vi "app - monitor RUS scan -- works.vi"(10 "normalize phase":bool) -> ()   [LabVIEW 2015]
uses:
  complex region.ctl
  lorentzian.ctl
  circle corners.ctl
  cursor winow.ctl
  scale - offset gauge.ctl
  <vilib>/event_ctls.llb/eventvkey.ctl
  peak -- parameters -- complex fit.ctl
  wavepacket.ctl
  filter method control.ctl
  parameters -- scan monitor control.ctl
  monitor state.ctl
  peak monitor ctl - V2.ctl
  interpolation state - real.ctl
  countdown control.ctl
  cursor window action.ctl
  plot refs -- filter related.ctl
  monitor action.ctl
  read scan file control.ctl
  ctl -- name dispatcher -- action.ctl
  Q -- check range -- i -- real - window.vi
  array -- find interval - real.vi
  next chunk - read-write freq PID file - atomic actions .vi
  Q -- check range -- i -- integer.vi
  aggregator - vi - real - atomic.vi
  switch - C.vi
  acquire cursor window data.vi
  filter - complex - four.vi
  peak -- PM find lorenzian - V2.vi
  linear interp iiii- complex - z-omega.vi
  line -- complex.vi
  Q - not nan -- real.vi
  array -- find index - real.vi
  array -- interpolate -- i.vi
  Q - not nan -- integer.vi
  linear interpolation - real.vi
  tale of three indices.vi
  filter -- window span logic.vi
  linear interp iiii- complex - z-omega - divide.vi
  linear interpolation iiii- complex.vi
  containing bix.vi
  peak -- guess at omega -- dzdomega.vi
  <vilib>/Analysis/baseanly.llb/A x B.vi
  <vilib>/Analysis/baseanly.llb/Complex A x B.vi
  command stack.vi
  tale of three indices -- check state.vi
  peak -- z center from mult phase points.vi
  peak -- estimate for lorentzian.vi
  peak -- fake phase around center.vi
  peak -- get weights.vi
  peak -- four corner circle transformation logic.vi
  peak - fit phase around center - V1.vi
  circle center from three points.vi
  <vilib>/Utility/error.llb/Clear Errors.vi
  <vilib>/Utility/libraryn.llb/Check if File or Folder Exists.vi
  file -- read list of lines.vi
  parse -- find first line.vi
  parse -- get list of matches -- numbers.vi
  <vilib>/Utility/file.llb/Write To Spreadsheet File (string).vi
  <vilib>/gmath/function.llb/Binomial Coefficient.vi
  monitor -- write section files.vi
  <vilib>/Analysis/Matrix/Numeric/Conversions/Array To Matrix.vi
  <vilib>/Analysis/Matrix/Numeric/Conversions/Array To Matrix - RA2.vi
  <vilib>/Analysis/baseanly.llb/Inverse Matrix.vi
  <vilib>/Analysis/baseanly.llb/Real Inverse Matrix.vi
  array - generate range.vi
  peak -- fit function -- arctan.vi
  <vilib>/gmath/NumericalOptimization/Nonlinear Curve Fit.vi
  <vilib>/gmath/NumericalOptimization/Nonlinear Curve Fit LM.vi
  filter pipe - plot staff - more - V2.vi
panel:
  out "current resonance #":i32
  in  "overwriting !!":bool
  in  "current resonance #":i32
  in  "overwrite (d)":enum16{"DUMP", "WORK", ""}(ring)
  in  "Tab : monitor":enum32{"main", "EDIT"}(tab)
  in  "scan monitor control":T1={"gamma acc. frac. - min "=0.3, "gamma acc frac.. - max"=3.0, "peak acc. fraction (af)"=5.0, "min peak acc. window (kHz)"=0.5, "use"=enum."fraction", "abs gamma min(kHz)"=0.005, "abs gamma max(kHz)"=5.0, "# points"=5, "gamma-factor (fa)"=5.0, "interpolate"=enum."line", "init"=TRUE, "Unique strike parameters"=TRUE, "max peak acc. window (kHz)"=10.0, "spacing factor"=1.5, "iterate #"=1, "overwrite ctl?"=FALSE, "write _m files?"=FALSE, "max slope (kHz/sweep)"=0.5, "funnel state"=enum."funnel open"}
  in  "monitor state":T2={"header - gamma"=[], "header - frequency"=[], "# of peaks"=32, "peaks OK"=FALSE}
  in  "autopilot":enum32{"on", "off"}(tab)=enum."off"
  in  "timer \"v\"":dbl(slide)=3.8370000000122673 min=-14768275.999999998 max=2129711151.0 step=0.01 scale=0.0..5.0 scale format="%#3_3f"
  in  "timer  \"update\"":dbl(slide)=3.8469999999961146 min=-14763200.0 max=2129711151.0 step=0.010000000000000002 scale=0.0..10.0 scale format="%#3_3f"
  in  "Temperature (K)":dbl=300.461
  in  "Magn Field (T)":dbl
  in  "Array of states":T3[](array[typedef])=[{"delta"=-0.0016575432837271364, "gamma"=0.76553, "exp"=652.9113, "found?"=TRUE, "found"=652.9096424567163, "gamma found"=0.7013829844109373, "init linear"=FALSE, "interpolate"=enum."line", "gamma-factor"=5.0, "slope"=-0.0044851701449078974, "update freq?"=TRUE, "update gamma?"=TRUE, "acc factor"=5.0, "linear interpolation state"={"requested size"=5, "Array"=[652.9241022479541, 652.9241022479541, 652.9081701289798, 652.9081701289798, 652.9096424567163], "actual number of elements"=5}, "ind"=0.0, "gamma ratio"=0.9162057455761854, "gamma off limit?"=FALSE, "freq off limit?"=FALSE}, {"delta"=0.003759118773814407, "gamma"=0.17466, "exp"=1036.47326, "found?"=TRUE, "found"=1036.4770191187738, "gamma found"=0.18203135700796666, "init linear"=FALSE, "interpolate"=enum."line", "gamma-factor"=5.0, "slope"=-0.0007907161774346605, "update freq?"=TRUE, "update gamma?"=TRUE, "acc factor"=5.0, "linear interpolation state"={"requested size"=5, "Array"=[1036.4789192628243, 1036.4789192628243, 1036.4748123891509, 1036.4748123891509, 1036.4770191187738], "actual number of elements"=5}, "ind"=1.0, "gamma ratio"=1.042204036459216, "gamma off limit?"=FALSE, "freq off limit?"=FALSE}, {"delta"=0.0049091040252733364, "gamma"=0.2876, "exp"=1456.4571, "found?"=TRUE, "found"=1456.4620091040254, "gamma found"=0.29018960202050387, "init linear"=FALSE, "interpolate"=enum."line", "gamma-factor"=5.0, "slope"=0.0005201884449343197, "update freq?"=TRUE, "update gamma?"=TRUE, "acc factor"=5.0, "linear interpolation state"={"requested size"=5, "Array"=[1456.4592147196108, 1456.4592147196108, 1456.4588278352328, 1456.4588278352328, 1456.4620091040254], "actual number of elements"=5}, "ind"=2.0, "gamma ratio"=1.0090041794871483, "gamma off limit?"=FALSE, "freq off limit?"=FALSE}, {"delta"=0.0007394967815343989, "gamma"=0.09637, "exp"=1508.93353, "found?"=TRUE, "found"=1508.9342694967816, "gamma found"=0.09651911838128847, "init linear"=FALSE, "interpolate"=enum."line", "gamma-factor"=5.0, "slope"=-0.00010129910398973152, "update freq?"=TRUE, "update gamma?"=TRUE, "acc factor"=5.0, "linear interpolation state"={"requested size"=5, "Array"=[1508.934330293854, 1508.934330293854, 1508.9334388969608, 1508.9334388969608, 1508.9342694967816], "actual number of elements"=5}, "ind"=3.0, "gamma ratio"=1.0015473527164935, "gamma off limit?"=FALSE, "freq off limit?"=FALSE}, {"delta"=-0.029278381005497067, "gamma"=0.50061, "exp"=1568.62295, "found?"=TRUE, "found"=1568.5936716189944, "gamma found"=0.29241762919205017, "init linear"=FALSE, "interpolate"=enum."line", "gamma-factor"=5.0, "slope"=0.002435031997738406, "update freq?"=TRUE, "update gamma?"=TRUE, "acc factor"=5.0, "linear interpolation state"={"requested size"=5, "Array"=[1568.5938152073131, 1568.5938152073131, 1568.618452703927, 1568.618452703927, 1568.5936716189944], "actual number of elements"=5}, "ind"=4.0, "gamma ratio"=0.5841226287769924, "gamma off limit?"=FALSE, "freq off limit?"=FALSE}, {"delta"=0.0026202347487469524, "gamma"=0.0806, "exp"=1635.60553, "found?"=TRUE, "found"=1635.6081502347488, "gamma found"=0.08233227541925552, "init linear"=FALSE, "interpolate"=enum."line", "gamma-factor"=5.0, "slope"=-0.0002922362121171318, "update freq?"=TRUE, "update gamma?"=TRUE, "acc factor"=5.0, "linear interpolation state"={"requested size"=5, "Array"=[1635.6087113801916, 1635.6087113801916, 1635.6069113089588, 1635.6069113089588, 1635.6081502347488], "actual number of elements"=5}, "ind"=5.0, "gamma ratio"=1.0214922508592494, "gamma off limit?"=FALSE, "freq off limit?"=FALSE}, {"delta"=-0.002563017279953783, "gamma"=0.23948, "exp"=1764.33943, "found?"=TRUE, "found"=1764.33686698272, "gamma found"=0.24236340731954384, "init linear"=FALSE, "interpolate"=enum."line", "gamma-factor"=5.0, "slope"=-0.0006999494679621421, "update freq?"=TRUE, "update gamma?"=TRUE, "acc factor"=5.0, "linear interpolation state"={"requested size"=5, "Array"=[1764.3399842040806, 1764.3399842040806, 1764.339219152121, 1764.339219152121, 1764.33686698272], "actual number of elements"=5}, "ind"=6.0, "gamma ratio"=1.012040284447736, "gamma off limit?"=FALSE, "freq off limit?"=FALSE}, {"delta"=0.0013207520305513754, "gamma"=0.09629, "exp"=2205.10687, "found?"=TRUE, "found"=2205.1081907520306, "gamma found"=0.0924387831546914, "init linear"=FALSE, "interpolate"=enum."line", "gamma-factor"=5.0, "slope"=-7.088923128321767e-05, "update freq?"=TRUE, "update gamma?"=TRUE, "acc factor"=5.0, "linear interpolation state"={"requested size"=5, "Array"=[2205.108115975172, 2205.108115975172, 2205.1072575291464, 2205.1072575291464, 2205.1081907520306], "actual number of elements"=5}, "ind"=7.0, "gamma ratio"=0.9600039791742797, "gamma off limit?"=FALSE, "freq off limit?"=FALSE}, {"delta"=0.003409232488138514, "gamma"=0.15471, "exp"=2247.57115, "found?"=TRUE, "found"=2247.5745592324884, "gamma found"=0.1527741784741036, "init linear"=FALSE, "interpolate"=enum."line", "gamma-factor"=5.0, "slope"=-0.0009672962635522708, "update freq?"=TRUE, "update gamma?"=TRUE, "acc factor"=5.0, "linear interpolation state"={"requested size"=5, "Array"=[2247.5776758034717, 2247.5776758034717, 2247.574235982803, 2247.574235982803, 2247.5745592324884], "actual number of elements"=5}, "ind"=8.0, "gamma ratio"=0.9874874182283214, "gamma off limit?"=FALSE, "freq off limit?"=FALSE}, {"delta"=-0.008548894449631916, "gamma"=0.16479, "exp"=2285.77663, "found?"=TRUE, "found"=2285.76808110555, "gamma found"=0.1267187147828005, "init linear"=FALSE, "interpolate"=enum."line", "gamma-factor"=5.0, "slope"=-0.0016395337344147264, "update freq?"=TRUE, "update gamma?"=TRUE, "acc factor"=5.0, "linear interpolation state"={"requested size"=5, "Array"=[2285.7766292086317, 2285.7766292086317, 2285.77733007745, 2285.77733007745, 2285.76808110555], "actual number of elements"=5}, "ind"=9.0, "gamma ratio"=0.7689709010425421, "gamma off limit?"=FALSE, "freq off limit?"=FALSE}, {"delta"=0.0004447395758688799, "gamma"=0.21964, "exp"=2405.10472, "found?"=TRUE, "found"=2405.1051647395757, "gamma found"=0.22044726667002684, "init linear"=FALSE, "interpolate"=enum."line", "gamma-factor"=5.0, "slope"=-0.0008384914183989168, "update freq?"=TRUE, "update gamma?"=TRUE, "acc factor"=5.0, "linear interpolation state"={"requested size"=5, "Array"=[2405.1081612139637, 2405.1081612139637, 2405.10576924856, 2405.10576924856, 2405.1051647395757], "actual number of elements"=5}, "ind"=10.0, "gamma ratio"=1.0036754082590915, "gamma off limit?"=FALSE, "freq off limit?"=FALSE}, {"delta"=0.0003001280488206248, "gamma"=0.22537, "exp"=2483.53635, "found?"=TRUE, "found"=2483.5366501280487, "gamma found"=0.2213622002178064, "init linear"=FALSE, "interpolate"=enum."line", "gamma-factor"=5.0, "slope"=-5.884840269573033e-05, "update freq?"=TRUE, "update gamma?"=TRUE, "acc factor"=5.0, "linear interpolation state"={"requested size"=5, "Array"=[2483.536882570466, 2483.536882570466, 2483.5367589712696, 2483.5367589712696, 2483.5366501280487], "actual number of elements"=5}, "ind"=11.0, "gamma ratio"=0.9822168000080153, "gamma off limit?"=FALSE, "freq off limit?"=FALSE}, {"delta"=-0.00047377254441016703, "gamma"=0.1374, "exp"=2613.48596, "found?"=TRUE, "found"=2613.4854862274556, "gamma found"=0.13919976502630776, "init linear"=FALSE, "interpolate"=enum."line", "gamma-factor"=5.0, "slope"=-0.0004374731567804702, "update freq?"=TRUE, "update gamma?"=TRUE, "acc factor"=5.0, "linear interpolation state"={"requested size"=5, "Array"=[2613.4871697330486, 2613.4871697330486, 2613.4861620126653, 2613.4861620126653, 2613.4854862274556], "actual number of elements"=5}, "ind"=12.0, "gamma ratio"=1.0130987265379023, "gamma off limit?"=FALSE, "freq off limit?"=FALSE}, {"delta"=-0.0014333203166643216, "gamma"=0.23275, "exp"=2775.83282, "found?"=TRUE, "found"=2775.8313866796834, "gamma found"=0.2800873248387451, "init linear"=FALSE, "interpolate"=enum."line", "gamma-factor"=5.0, "slope"=9.053546469658613e-05, "update freq?"=TRUE, "update gamma?"=TRUE, "acc factor"=5.0, "linear interpolation state"={"requested size"=5, "Array"=[2775.8316113301, 2775.8316113301, 2775.8329659855785, 2775.8329659855785, 2775.8313866796834], "actual number of elements"=5}, "ind"=13.0, "gamma ratio"=1.2033827060740927, "gamma off limit?"=FALSE, "freq off limit?"=FALSE}, {"delta"=0.001513914386578108, "gamma"=0.0716, "exp"=2886.62499, "found?"=TRUE, "found"=2886.6265039143864, "gamma found"=0.07112662438840253, "init linear"=FALSE, "interpolate"=enum."line", "gamma-factor"=5.0, "slope"=-0.0006266225839499384, "update freq?"=TRUE, "update gamma?"=TRUE, "acc factor"=5.0, "linear interpolation state"={"requested size"=5, "Array"=[2886.628416499212, 2886.628416499212, 2886.6259754430316, 2886.6259754430316, 2886.6265039143864], "actual number of elements"=5}, "ind"=14.0, "gamma ratio"=0.9933886087765718, "gamma off limit?"=FALSE, "freq off limit?"=FALSE}, {"delta"=0.006262894615701953, "gamma"=0.14682, "exp"=2925.52376, "found?"=TRUE, "found"=2925.5300228946157, "gamma found"=0.14212049264176846, "init linear"=FALSE, "interpolate"=enum."line", "gamma-factor"=5.0, "slope"=-0.0013607249583583326, "update freq?"=TRUE, "update gamma?"=TRUE, "acc factor"=5.0, "linear interpolation state"={"requested size"=5, "Array"=[2925.5337999193525, 2925.5337999193525, 2925.5277467192377, 2925.5277467192377, 2925.5300228946157], "actual number of elements"=5}, "ind"=15.0, "gamma ratio"=0.9679913679455691, "gamma off limit?"=FALSE, "freq off limit?"=FALSE}, {"delta"=0.0008407358172917156, "gamma"=0.05724, "exp"=2968.74884, "found?"=TRUE, "found"=2968.7496807358175, "gamma found"=0.056604877858379594, "init linear"=FALSE, "interpolate"=enum."line", "gamma-factor"=5.0, "slope"=6.453693960793316e-05, "update freq?"=TRUE, "update gamma?"=TRUE, "acc factor"=5.0, "linear interpolation state"={"requested size"=5, "Array"=[2968.7492258726284, 2968.7492258726284, 2968.7489615156423, 2968.7489615156423, 2968.7496807358175], "actual number of elements"=5}, "ind"=16.0, "gamma ratio"=0.9889042253385674, "gamma off limit?"=FALSE, "freq off limit?"=FALSE}, {"delta"=0.0004893467435067578, "gamma"=0.18507, "exp"=3117.27562, "found?"=TRUE, "found"=3117.2761093467434, "gamma found"=0.18508310581473786, "init linear"=FALSE, "interpolate"=enum."line", "gamma-factor"=5.0, "slope"=-0.000674382079159841, "update freq?"=TRUE, "update gamma?"=TRUE, "acc factor"=5.0, "linear interpolation state"={"requested size"=5, "Array"=[3117.278479994366, 3117.278479994366, 3117.27647746882, 3117.27647746882, 3117.2761093467434], "actual number of elements"=5}, "ind"=17.0, "gamma ratio"=1.0000708154467923, "gamma off limit?"=FALSE, "freq off limit?"=FALSE}, {"delta"=0.0009432243264200224, "gamma"=0.11467, "exp"=3141.4319, "found?"=TRUE, "found"=3141.4328432243265, "gamma found"=0.11506466086057514, "init linear"=FALSE, "interpolate"=enum."line", "gamma-factor"=5.0, "slope"=-0.0002722086093854159, "update freq?"=TRUE, "update gamma?"=TRUE, "acc factor"=5.0, "linear interpolation state"={"requested size"=5, "Array"=[3141.4337316093643, 3141.4337316093643, 3141.432786293347, 3141.432786293347, 3141.4328432243265], "actual number of elements"=5}, "ind"=18.0, "gamma ratio"=1.0034417097808943, "gamma off limit?"=FALSE, "freq off limit?"=FALSE}, {"delta"=0.006890674223541282, "gamma"=0.19401, "exp"=3268.65403, "found?"=TRUE, "found"=3268.6609206742237, "gamma found"=0.1947000973954296, "init linear"=FALSE, "interpolate"=enum."line", "gamma-factor"=5.0, "slope"=0.001370561413350515, "update freq?"=TRUE, "update gamma?"=TRUE, "acc factor"=5.0, "linear interpolation state"={"requested size"=5, "Array"=[3268.654487682439, 3268.654487682439, 3268.6553273130035, 3268.6553273130035, 3268.6609206742237], "actual number of elements"=5}, "ind"=19.0, "gamma ratio"=1.0035570197176928, "gamma off limit?"=FALSE, "freq off limit?"=FALSE}, {"delta"=-0.00036122355459156097, "gamma"=0.09375, "exp"=3447.74234, "found?"=TRUE, "found"=3447.741978776445, "gamma found"=0.09343849466512388, "init linear"=FALSE, "interpolate"=enum."line", "gamma-factor"=5.0, "slope"=-0.0002539216459263116, "update freq?"=TRUE, "update gamma?"=TRUE, "acc factor"=5.0, "linear interpolation state"={"requested size"=5, "Array"=[3447.7428802682552, 3447.7428802682552, 3447.742144035429, 3447.742144035429, 3447.741978776445], "actual number of elements"=5}, "ind"=20.0, "gamma ratio"=0.9966772764279881, "gamma off limit?"=FALSE, "freq off limit?"=FALSE}, {"delta"=-3486.5123, "gamma"=0.01485, "exp"=3486.5123, "found?"=FALSE, "found"=0.0, "gamma found"=0.0, "init linear"=TRUE, "interpolate"=enum."line", "gamma-factor"=5.0, "slope"=0.0, "update freq?"=FALSE, "update gamma?"=FALSE, "acc factor"=5.0, "linear interpolation state"={"requested size"=5, "Array"=[0.0, 0.0, 0.0, 0.0, 3486.5122984940626], "actual number of elements"=1}, "ind"=21.0, "gamma ratio"=0.0, "gamma off limit?"=TRUE, "freq off limit?"=TRUE}, {"delta"=0.005188108485072007, "gamma"=0.2862, "exp"=3737.75053, "found?"=TRUE, "found"=3737.755718108485, "gamma found"=0.25947921890028686, "init linear"=FALSE, "interpolate"=enum."line", "gamma-factor"=5.0, "slope"=-0.0006564744841307402, "update freq?"=TRUE, "update gamma?"=TRUE, "acc factor"=5.0, "linear interpolation state"={"requested size"=5, "Array"=[3737.7568178710067, 3737.7568178710067, 3737.752452651206, 3737.752452651206, 3737.755718108485], "actual number of elements"=5}, "ind"=22.0, "gamma ratio"=0.9066359849765439, "gamma off limit?"=FALSE, "freq off limit?"=FALSE}, {"delta"=0.05791749378431632, "gamma"=0.1209, "exp"=3773.78708, "found?"=FALSE, "found"=3773.8449974937844, "gamma found"=0.0018969298658040622, "init linear"=FALSE, "interpolate"=enum."line", "gamma-factor"=7.0, "slope"=-0.027493364620750072, "update freq?"=TRUE, "update gamma?"=TRUE, "acc factor"=7.0, "linear interpolation state"={"requested size"=5, "Array"=[0.0, 3773.880271706499, 3773.8206547185614, 3773.825284977259, 3773.7870837381997], "actual number of elements"=4}, "ind"=23.0, "gamma ratio"=0.015690073331712674, "gamma off limit?"=TRUE, "freq off limit?"=FALSE}, {"delta"=0.0016448427732029813, "gamma"=0.14541, "exp"=4176.53307, "found?"=TRUE, "found"=4176.534714842774, "gamma found"=0.14055145401454877, "init linear"=FALSE, "interpolate"=enum."line", "gamma-factor"=5.0, "slope"=0.001082140458165668, "update freq?"=TRUE, "update gamma?"=TRUE, "acc factor"=5.0, "linear interpolation state"={"requested size"=5, "Array"=[4176.530918624351, 4176.530918624351, 4176.534147592093, 4176.534147592093, 4176.534714842774], "actual number of elements"=5}, "ind"=24.0, "gamma ratio"=0.9665872636995307, "gamma off limit?"=FALSE, "freq off limit?"=FALSE}, {"delta"=0.006093070963288483, "gamma"=0.07631, "exp"=4238.40966, "found?"=TRUE, "found"=4238.415753070964, "gamma found"=0.07370934433890397, "init linear"=FALSE, "interpolate"=enum."line", "gamma-factor"=5.0, "slope"=-0.0001927513594273478, "update freq?"=TRUE, "update gamma?"=TRUE, "acc factor"=5.0, "linear interpolation state"={"requested size"=5, "Array"=[4238.415194475135, 4238.415194475135, 4238.412149769886, 4238.412149769886, 4238.415753070964], "actual number of elements"=5}, "ind"=25.0, "gamma ratio"=0.9659198576713925, "gamma off limit?"=FALSE, "freq off limit?"=FALSE}, {"delta"=0.0014712240090375417, "gamma"=0.10797, "exp"=4931.57573, "found?"=TRUE, "found"=4931.577201224009, "gamma found"=0.1106825599113035, "init linear"=FALSE, "interpolate"=enum."line", "gamma-factor"=5.0, "slope"=0.0010064907773630694, "update freq?"=TRUE, "update gamma?"=TRUE, "acc factor"=5.0, "linear interpolation state"={"requested size"=5, "Array"=[4931.573629158262, 4931.573629158262, 4931.5765499345425, 4931.5765499345425, 4931.577201224009], "actual number of elements"=5}, "ind"=26.0, "gamma ratio"=1.0251232741622998, "gamma off limit?"=FALSE, "freq off limit?"=FALSE}, {"delta"=0.01094153662052122, "gamma"=0.05188, "exp"=5475.82656, "found?"=TRUE, "found"=5475.837501536621, "gamma found"=0.11863591544266465, "init linear"=FALSE, "interpolate"=enum."line", "gamma-factor"=8.0, "slope"=0.0012847163761034609, "update freq?"=TRUE, "update gamma?"=TRUE, "acc factor"=8.0, "linear interpolation state"={"requested size"=5, "Array"=[5475.831455900791, 5475.831455900791, 5475.832211792886, 5475.832211792886, 5475.837501536621], "actual number of elements"=5}, "ind"=27.0, "gamma ratio"=2.2867369977383314, "gamma off limit?"=FALSE, "freq off limit?"=FALSE}, {"delta"=-5768.35916, "gamma"=0.005, "exp"=5768.35916, "found?"=FALSE, "found"=0.0, "gamma found"=0.0, "init linear"=TRUE, "interpolate"=enum."line", "gamma-factor"=5.0, "slope"=0.0, "update freq?"=FALSE, "update gamma?"=FALSE, "acc factor"=5.0, "linear interpolation state"={"requested size"=5, "Array"=[0.0, 0.0, 0.0, 0.0, 5768.359158074293], "actual number of elements"=1}, "ind"=28.0, "gamma ratio"=0.0, "gamma off limit?"=TRUE, "freq off limit?"=TRUE}, {"delta"=18.256138418231785, "gamma"=0.02905, "exp"=6148.70194, "found?"=FALSE, "found"=6166.958078418232, "gamma found"=4.5314912463139816e-05, "init linear"=TRUE, "interpolate"=enum."line", "gamma-factor"=5.0, "slope"=0.0, "update freq?"=FALSE, "update gamma?"=FALSE, "acc factor"=5.0, "linear interpolation state"={"requested size"=5, "Array"=[0.0, 0.0, 0.0, 0.0, 6148.701943422434], "actual number of elements"=1}, "ind"=29.0, "gamma ratio"=0.001559893716459202, "gamma off limit?"=TRUE, "freq off limit?"=TRUE}, {"delta"=0.004358224254247034, "gamma"=0.0424, "exp"=5751.24344, "found?"=TRUE, "found"=5751.247798224254, "gamma found"=0.0686871247901866, "init linear"=TRUE, "interpolate"=enum."line", "gamma-factor"=7.0, "slope"=0.0, "update freq?"=FALSE, "update gamma?"=FALSE, "acc factor"=7.0, "linear interpolation state"={"requested size"=5, "Array"=[0.0, 0.0, 0.0, 0.0, 5751.24344], "actual number of elements"=1}, "ind"=30.0, "gamma ratio"=1.619979358259118, "gamma off limit?"=FALSE, "freq off limit?"=FALSE}, {"delta"=0.02459476473813993, "gamma"=0.14229, "exp"=6300.95565, "found?"=TRUE, "found"=6300.980244764738, "gamma found"=0.1593322314931949, "init linear"=FALSE, "interpolate"=enum."line", "gamma-factor"=7.0, "slope"=0.001076212803600356, "update freq?"=TRUE, "update gamma?"=TRUE, "acc factor"=7.0, "linear interpolation state"={"requested size"=5, "Array"=[6300.9711810739645, 6300.9711810739645, 6300.963815820454, 6300.963815820454, 6300.980244764738], "actual number of elements"=5}, "ind"=31.0, "gamma ratio"=1.1197711117660756, "gamma off limit?"=FALSE, "freq off limit?"=FALSE}]
  in  "dump/work NEW (\"n\")":enum16{"DUMP", "WORK", ""}(ring)
  in  "NEW freq":dbl[](array[numeric])=[652.901381931682, 1036.4745243360126, 1456.4611794080774, 1508.93365767837, 1568.6109465842878, 1635.607002413974, 1764.33695489062, 2205.1075748844396, 2247.5727746722177, 2285.770281334339, 2405.104089658669, 2483.536610097096, 2613.485117524306, 2775.8323798686024, 2886.625177692022, 2925.5265410594843, 2968.74940471329, 3117.275181708386, 3141.432359180121, 3268.6602218172616, 3447.7416437118245, 3486.5122984940626, 3737.7528824071287, 3773.7595903735782, 4176.536215876507, 4238.4135100581225, 4931.5785313542565, 5475.8368215339215, 5768.359158074293, 6148.701943422434, 5751.24344, 6300.973276349126]
  in  "NEW gamma":dbl[](array[numeric])=[0.7013829844109373, 0.18203135700796666, 0.29018960202050387, 0.09651911838128847, 0.29241762919205017, 0.08233227541925552, 0.24236340731954384, 0.0924387831546914, 0.1527741784741036, 0.1267187147828005, 0.22044726667002684, 0.2213622002178064, 0.13919976502630776, 0.2800873248387451, 0.07112662438840253, 0.14212049264176846, 0.056604877858379594, 0.18508310581473786, 0.11506466086057514, 0.1947000973954296, 0.09343849466512388, 0.01485, 0.25947921890028686, 0.1209, 0.14055145401454877, 0.07370934433890397, 0.1106825599113035, 0.11863591544266465, 0.005, 0.02905, 0.0424, 0.1593322314931949]
  in  "OLD gamma":dbl[](array[numeric])
  in  "OLD freq":dbl[](array[numeric])
  out "cp lorentzian":T5={"Amplitude"=0.000340055891053764, "omega(0)"=3392.560000065714, "Gamma"=11.91999763250351, "phase"=1.0574274315248449, "Q"=284.61079478865537, "Norm  Ampl"=nan, "z (inf)"=-2.2995916620324662e-05-1.1031702558117846e-05i, "4corners"={"z (-pi/2)"=1.5865449989673634e-05-1.9155492294065609e-07i, "z(inf)"=-2.2995916620324662e-05-1.1031702558117846e-05i, "z (pi/2)"=-1.2155768985147472e-05-4.9893069168116145e-05i, "z center"=1.8548405022630806e-06-2.50423120455284e-05i, "z(0)"=2.6705597624850824e-05-3.905292153293895e-05i, "radius"=2.8528184445817156e-05}} {"z (inf)" format="%#9_9f"; "Q" format="%#9_9f"; "phase" format="%#9_9f"; "Gamma" format="%#9_9f"; "omega(0)" format="%#9_9f"}
  out "index":i32[](array[numeric])=[0, 1, 2, 3, 4, 5, 6, 7, 8, 9, 10, 11, 12, 13, 14, 15, 16, 17, 18, 19, 20, 21, 22, 23, 24, 25, 26, 27, 28, 29, 30, 31, 32, 33, 34, 35, 36, 37, 38, 39, 40, 41, 42, 43, 44, 45, 46, 47, 48, 49, 50, 51, 52, 53, 54, 55, 56, 57, 58, 59, 60, 61, 62, 63, 64, 65, 66, 67, 68, 69, 70, 71, 72, 73, 74, 75, 76, 77, 78, 79, 80, 81, 82, 83, 84, 85, 86, 87, 88, 89, 90, 91, 92, 93, 94, 95, 96, 97, 98, 99]
  in  "Tab : everything":T7(tab)
  in  "Tab :  Fit controls":enum32{"complex plane", "complex plane 2"}(tab)
  in  "Plot: fragment - filter":cluster{dbl[], dbl[]}[](graph)=[{array[953 elements], array[953 elements]}, {array[953 elements], array[953 elements]}, {array[953 elements], array[953 elements]}, {array[953 elements], array[953 elements]}]
  in  "scale gauge: Plot: complex plane - filter":dbl(slide)=0.00199 min=0.0 max=0.3 step=1e-05 scale=0.0001..0.3 scale format="%#_5g"
  in  "Plot: complex plane - filter":cluster{dbl[], dbl[]}[](graph)=[{array[953 elements], array[953 elements]}, {array[953 elements], array[953 elements]}, {[6.147901040838566e-05, 6.135373133876665e-05, 6.097838854916284e-05, 6.0354463346086974e-05, 5.948441807727129e-05, 5.837168641390595e-05, 5.702065979950748e-05, 5.54366701188976e-05, 5.362596865568959e-05, 5.1595701421327945e-05, 4.9353880953045816e-05, 4.690935469204115e-05, 4.427177006666834e-05, 4.145153641844591e-05, 3.8459783921141216e-05, 3.5308319655059415e-05, 3.200958100989166e-05, 2.8576586600020083e-05, 2.5022884885994518e-05, 2.1362500704948304e-05, 1.7609879920973602e-05, 1.3779832413895373e-05, 9.887473631441806e-06, 5.948164935477676e-06, 1.9774529777269755e-06, -2.0089916557587785e-06, -5.995436289244519e-06, -9.96614824699522e-06, -1.3905456942959363e-05, -1.779781572541292e-05, -2.1627863232491146e-05, -2.5380484016465848e-05, -2.904086819751206e-05, -3.259456991153764e-05, -3.6027564321409215e-05, -3.932630296657695e-05, -4.247776723265876e-05, -4.5469519729963454e-05, -4.8289753378185884e-05, -5.09273380035587e-05, -5.3371864264563346e-05, -5.561368473284548e-05, -5.764395196720713e-05, -5.945465343041514e-05, -6.103864311102503e-05, -6.238966972542349e-05, -6.350240138878883e-05, -6.437244665760451e-05, -6.499637186068038e-05, -6.537171465028419e-05, -6.54969937199032e-05, -6.537171465028419e-05, -6.499637186068038e-05, -6.437244665760451e-05, -6.350240138878883e-05, -6.238966972542349e-05, -6.103864311102501e-05, -5.945465343041513e-05, -5.764395196720712e-05, -5.5613684732845474e-05, -5.337186426456334e-05, -5.092733800355868e-05, -4.828975337818588e-05, -4.546951972996345e-05, -4.2477767232658746e-05, -3.9326302966576966e-05, -3.602756432140918e-05, -3.2594569911537626e-05, -2.904086819751202e-05, -2.5380484016465838e-05, -2.1627863232491146e-05, -1.7797815725412892e-05, -1.390545694295935e-05, -9.966148246995179e-06, -5.995436289244506e-06, -2.0089916557587802e-06, 1.9774529777270017e-06, 5.9481649354776745e-06, 9.887473631441845e-06, 1.3779832413895386e-05, 1.760987992097359e-05, 2.1362500704948328e-05, 2.5022884885994515e-05, 2.8576586600020124e-05, 3.200958100989167e-05, 3.5308319655059456e-05, 3.8459783921141236e-05, 4.145153641844591e-05, 4.427177006666836e-05, 4.690935469204116e-05, 4.9353880953045836e-05, 5.159570142132796e-05, 5.362596865568959e-05, 5.543667011889761e-05, 5.702065979950749e-05, 5.837168641390596e-05, 5.9484418077271304e-05, 6.0354463346086974e-05, 6.097838854916284e-05, 6.135373133876665e-05], [-1.1205323218261426e-05, -7.218878584775678e-06, -3.2481666270249814e-06, 6.911420689391552e-07, 4.583500851392718e-06, 8.413548358470941e-06, 1.2166169142445653e-05, 1.5826553323491864e-05, 1.938025503751744e-05, 2.2813249447389007e-05, 2.6111988092556765e-05, 2.9263452358638565e-05, 3.225520485594326e-05, 3.507543850416568e-05, 3.7713023129538496e-05, 4.015754939054316e-05, 4.239936985882529e-05, 4.442963709318694e-05, 4.6240338556394946e-05, 4.782432823700483e-05, 4.917535485140329e-05, 5.028808651476863e-05, 5.115813178358432e-05, 5.178205698666018e-05, 5.2157399776263995e-05, 5.2282678845883e-05, 5.2157399776263995e-05, 5.178205698666017e-05, 5.115813178358432e-05, 5.028808651476863e-05, 4.917535485140329e-05, 4.7824328237004825e-05, 4.624033855639494e-05, 4.4429637093186926e-05, 4.239936985882528e-05, 4.015754939054316e-05, 3.7713023129538496e-05, 3.5075438504165676e-05, 3.2255204855943246e-05, 2.926345235863855e-05, 2.611198809255677e-05, 2.2813249447389007e-05, 1.9380255037517432e-05, 1.5826553323491847e-05, 1.216616914244564e-05, 8.413548358470924e-06, 4.583500851392722e-06, 6.911420689391518e-07, -3.2481666270249915e-06, -7.218878584775692e-06, -1.1205323218261446e-05, -1.5191767851747172e-05, -1.9162479809497872e-05, -2.3101788505462016e-05, -2.6994147287915587e-05, -3.082419479499382e-05, -3.4576815578968526e-05, -3.8237199760014716e-05, -4.179090147404029e-05, -4.5223895883911866e-05, -4.852263452907963e-05, -5.167409879516143e-05, -5.466585129246611e-05, -5.7486084940688535e-05, -6.0123669566061355e-05, -6.2568195827066e-05, -6.481001629534815e-05, -6.684028352970978e-05, -6.865098499291781e-05, -7.023497467352768e-05, -7.158600128792615e-05, -7.26987329512915e-05, -7.356877822010717e-05, -7.419270342318303e-05, -7.456804621278685e-05, -7.469332528240585e-05, -7.456804621278685e-05, -7.419270342318303e-05, -7.356877822010717e-05, -7.269873295129148e-05, -7.158600128792615e-05, -7.023497467352767e-05, -6.86509849929178e-05, -6.684028352970978e-05, -6.481001629534813e-05, -6.256819582706598e-05, -6.0123669566061334e-05, -5.7486084940688535e-05, -5.4665851292466084e-05, -5.167409879516141e-05, -4.8522634529079576e-05, -4.522389588391184e-05, -4.179090147404029e-05, -3.823719976001468e-05, -3.45768155789685e-05, -3.0824194794993756e-05, -2.6994147287915553e-05, -2.310178850546201e-05, -1.9162479809497842e-05, -1.5191767851747167e-05]}, {[2.180843613001339e-05, -2.008991706602334e-06, -8.45318187396811e-06], [2.015688719802568e-05, -1.1205323149030123e-05, 1.4773194307782804e-05]}, {[3.113757403751932e-06, 2.0471841396985487e-06, 9.806108756451657e-07, -8.596238840821741e-08, -1.1525356524616005e-06, -2.2191089165149835e-06, -3.2856821805683666e-06, -4.35225544462175e-06, -5.418828708675133e-06, -6.485401972728517e-06, -7.551975236781899e-06, -8.618548500835281e-06, -9.685121764888665e-06, -1.0751695028942049e-05, -1.1818268292995431e-05, -1.2884841557048813e-05, -1.3951414821102197e-05, -1.5017988085155581e-05, -1.6084561349208965e-05, -1.7151134613262346e-05], [7.143908232533313e-06, 6.9167218796742506e-06, 6.689535526815188e-06, 6.462349173956126e-06, 6.235162821097064e-06, 6.0079764682380015e-06, 5.780790115378939e-06, 5.553603762519877e-06, 5.326417409660815e-06, 5.0992310568017525e-06, 4.87204470394269e-06, 4.644858351083628e-06, 4.417671998224566e-06, 4.1904856453655035e-06, 3.963299292506441e-06, 3.736112939647379e-06, 3.5089265867883167e-06, 3.2817402339292544e-06, 3.054553881070192e-06, 2.82736752821113e-06]}, {[-2.0089917066023344e-06, -9.360762157193256e-07, 1.3683927516368315e-07, 1.2097547660466921e-06, 2.2826702569297007e-06, 3.3555857478127092e-06, 4.428501238695719e-06, 5.501416729578727e-06, 6.574332220461736e-06, 7.647247711344744e-06, 8.720163202227753e-06, 9.793078693110761e-06, 1.0865994183993772e-05, 1.193890967487678e-05, 1.3011825165759789e-05, 1.4084740656642797e-05, 1.5157656147525806e-05, 1.6230571638408814e-05, 1.7303487129291823e-05, 1.837640262017483e-05], [-1.1205323149030123e-05, -1.1205323149030123e-05, -1.1205323149030123e-05, -1.1205323149030123e-05, -1.1205323149030123e-05, -1.1205323149030123e-05, -1.1205323149030123e-05, -1.1205323149030123e-05, -1.1205323149030123e-05, -1.1205323149030123e-05, -1.1205323149030123e-05, -1.1205323149030123e-05, -1.1205323149030123e-05, -1.1205323149030123e-05, -1.1205323149030123e-05, -1.1205323149030123e-05, -1.1205323149030123e-05, -1.1205323149030123e-05, -1.1205323149030123e-05, -1.1205323149030123e-05]}]
  out "Plot: dz/domega":cluster{"omega out":dbl[], dbl[]}(graph)
  out "Plot: win omega":T8(graph)
  out "Plot: phase":cluster{"omega out":dbl[], dbl[]}(graph)
  out "Plot: phase around center":cluster{dbl[], dbl[]}[](graph)
  out "Plot: fragment":cluster{dbl[], dbl[]}[](graph)
  out "Plot: complex plane":cluster{dbl[], dbl[]}[](graph)=[{array[953 elements], array[953 elements]}, {[3.0383024948080237e-05, 3.01580716927693e-05, 2.9486759574053305e-05, 2.8379675585066826e-05, 2.68542791016561e-05, 2.4934626537592202e-05, 2.2650991960555277e-05, 2.0039389652002364e-05, 1.714100614043495e-05, 1.4001550665240835e-05, 1.0670534314683625e-05, 7.200489206464318e-06, 3.646140024844015e-06, 6.354097968214359e-08, -3.4908082019381657e-06, -6.960853310157466e-06, -1.0291869660714675e-05, -1.3431325135908794e-05, -1.6329708647476206e-05, -1.8941310956029118e-05, -2.1224945533066037e-05, -2.314459809712994e-05, -2.4669994580540667e-05, -2.5777078569527143e-05, -2.6448390688243138e-05, -2.6673343943554075e-05, -2.6448390688243138e-05, -2.5777078569527143e-05, -2.466999458054066e-05, -2.3144598097129935e-05, -2.1224945533066034e-05, -1.8941310956029115e-05, -1.63297086474762e-05, -1.343132513590878e-05, -1.0291869660714658e-05, -6.960853310157466e-06, -3.49080820193816e-06, 6.354097968214909e-08, 3.646140024844027e-06, 7.200489206464335e-06, 1.0670534314683618e-05, 1.4001550665240833e-05, 1.7141006140434956e-05, 2.003938965200237e-05, 2.2650991960555284e-05, 2.4934626537592213e-05, 2.68542791016561e-05, 2.837967558506683e-05, 2.948675957405331e-05, 3.01580716927693e-05], [-2.50423120455284e-05, -2.1466782441215247e-05, -1.7947641074679964e-05, -1.454038690750597e-05, -1.1298754373304577e-05, -8.273865953597556e-06, -5.513425945744431e-06, -3.060968137675989e-06, -9.551692540527458e-07, 7.707609987872854e-07, 2.0896036697360487e-06, 2.9805598220342752e-06, 3.429578544928799e-06, 3.429578544928799e-06, 2.980559822034272e-06, 2.0896036697360487e-06, 7.70760998787282e-07, -9.551692540527492e-07, -3.060968137675989e-06, -5.513425945744438e-06, -8.273865953597552e-06, -1.129875437330458e-05, -1.4540386907505977e-05, -1.7947641074679964e-05, -2.146678244121525e-05, -2.504231204552841e-05, -2.8617841649841554e-05, -3.213698301637684e-05, -3.554423718355084e-05, -3.878586971775222e-05, -4.1810758137459246e-05, -4.4571198145312364e-05, -4.702365595338081e-05, -4.912945483700406e-05, -5.085538508984409e-05, -5.217422776079284e-05, -5.3065183913091077e-05, -5.35142026359856e-05, -5.35142026359856e-05, -5.306518391309107e-05, -5.217422776079285e-05, -5.085538508984409e-05, -4.912945483700405e-05, -4.7023655953380806e-05, -4.457119814531235e-05, -4.181075813745923e-05, -3.878586971775222e-05, -3.5544237183550826e-05, -3.213698301637683e-05, -2.8617841649841537e-05]}, {[-2.2995916620324662e-05, -2.051084090806589e-05, -1.8025765195807113e-05, -1.554068948354834e-05, -1.3055613771289565e-05, -1.057053805903079e-05, -8.085462346772018e-06, -5.600386634513241e-06, -3.1153109222544683e-06, -6.302352099956953e-07, 1.854840502263081e-06, 4.339916214521854e-06, 6.824991926780627e-06, 9.310067639039403e-06, 1.179514335129818e-05, 1.4280219063556949e-05, 1.6765294775815725e-05, 1.92503704880745e-05, 2.173544620033327e-05, 2.4220521912592048e-05], [-1.1031702558117846e-05, -1.2432763506858901e-05, -1.3833824455599956e-05, -1.5234885404341013e-05, -1.6635946353082066e-05, -1.8037007301823124e-05, -1.943806825056418e-05, -2.0839129199305234e-05, -2.224019014804629e-05, -2.3641251096787344e-05, -2.50423120455284e-05, -2.6443372994269454e-05, -2.7844433943010512e-05, -2.9245494891751567e-05, -3.064655584049262e-05, -3.2047616789233674e-05, -3.344867773797473e-05, -3.484973868671579e-05, -3.625079963545684e-05, -3.7651860584197894e-05]}, {[1.5865449989673634e-05, 1.4464389040932579e-05, 1.3063328092191524e-05, 1.1662267143450467e-05, 1.0261206194709412e-05, 8.860145245968358e-06, 7.459084297227301e-06, 6.058023348486246e-06, 4.656962399745191e-06, 3.255901451004136e-06, 1.854840502263081e-06, 4.5377955352202603e-07, -9.472813952190323e-07, -2.3483423439600873e-06, -3.7494032927011422e-06, -5.150464241442197e-06, -6.551525190183252e-06, -7.952586138924307e-06, -9.353647087665362e-06, -1.0754708036406417e-05], [-1.9155492294065947e-07, -2.6766306351994337e-06, -5.161706347458208e-06, -7.646782059716982e-06, -1.0131857771975756e-05, -1.2616933484234531e-05, -1.5102009196493304e-05, -1.758708490875208e-05, -2.0072160621010853e-05, -2.2557236333269626e-05, -2.5042312045528402e-05, -2.7527387757787175e-05, -3.0012463470045948e-05, -3.2497539182304725e-05, -3.49826148945635e-05, -3.746769060682227e-05, -3.995276631908105e-05, -4.243784203133982e-05, -4.492291774359859e-05, -4.740799345585737e-05]}, {[0.04673210164257447, 0.049919815487102684, 0.05307633107191166, 0.056199675677509844, 0.05928789731518806, 0.06233906594694866, 0.06535127469171664, 0.06832264101707818, 0.07125130791580202, 0.0741354450664087, 0.07697324997706184, 0.07976294911206679, 0.0825027990002728, 0.0851910873246857, 0.08782613399261033, 0.09040629218565366, 0.09292994938893286, 0.09539552839884442, 0.09780148830876523, 0.10014632547206899], [-0.12810601858774873, -0.1268978066952708, -0.12561028780431027, -0.1242442665722635, -0.12280059671793454, -0.12128018048798891, -0.11968396809307863, -0.11801295711399153, -0.11626819187819583, -0.11445076280716932, -0.11256180573492151, -0.11060250119813439, -0.10857407369836529, -0.10647779093677343, -0.10431496302184781, -0.10208694165063226, -0.09979511926395848, -0.09744092817621612, -0.09502583968020283, -0.09255136312761404]}, {[0.05358614321681127, 0.05724138842520362, 0.06086085962911791, 0.0644422947768705, 0.06798345558807486, 0.07148212895249367, 0.07493612831316095, 0.07834329503290884, 0.08170149974344551, 0.08500864367614118, 0.08826265997369011, 0.09146151498182913, 0.09460320952030535, 0.09768578013229881, 0.10070730031151905, 0.10366588170620873, 0.1065596752993022, 0.1093868725640008, 0.11214570659404333, 0.11483445320796498], [-0.1468949013139417, -0.145509485010567, -0.14403313001559898, -0.142466759002852, -0.14081135090322142, -0.13906794029288377, -0.13723761674671997, -0.13532152415736678, -0.13332086002032104, -0.13123687468554396, -0.12907087057603317, -0.1268242013738506, -0.12449827117411537, -0.12209453360749002, -0.11961449093170867, -0.11705969309271483, -0.11443173675599556, -0.11173226430871766, -0.10896296283328909, -0.10612556305298726]}, {array[953 elements], array[953 elements]}]
  in  "scale gauge: Plot: complex plane":dbl(slide)=0.08418000000000002 min=0.0 max=0.3 step=1e-05 scale=0.0001..1.0 scale format="%#_2g"
  in  "plot staff":enum16{"plot", "do not plot", "a"}(ring)=enum."do not plot"
  out "pm lorentzian":T5={"Amplitude"=0.000340055891053764, "omega(0)"=3392.560000065714, "Gamma"=11.91999763250351, "phase"=1.0574274315248449, "Q"=284.61079478865537, "Norm  Ampl"=nan, "z (inf)"=-2.2995916620324662e-05-1.1031702558117846e-05i, "4corners"={"z (-pi/2)"=1.5865449989673634e-05-1.9155492294065609e-07i, "z(inf)"=-2.2995916620324662e-05-1.1031702558117846e-05i, "z (pi/2)"=-1.2155768985147472e-05-4.9893069168116145e-05i, "z center"=1.8548405022630806e-06-2.50423120455284e-05i, "z(0)"=2.6705597624850824e-05-3.905292153293895e-05i, "radius"=2.8528184445817156e-05}} {"z (inf)" format="%#9_9f"; "Q" format="%#9_9f"; "phase" format="%#9_9f"; "Gamma" format="%#9_9f"; "omega(0)" format="%#9_9f"}
  in  "use fast fit?":bool=TRUE
  out "window width (kHz)":dbl=76.27809365793496
  out "window center (kHz)":dbl=3399.029286744401
  out "# of points in window":dbl=953.475933538175
  in  "Tab : all plot":enum32{"Page 1"}(tab)
  in  "scale gauge : All plot":T9={"scale offset"=0.5005000000000001, "scale range"=0.019950000000000002} {"scale range" min=0.0 max=1.0 step=1e-05 scale=0.001..1.0 scale format="%#_2g"; "scale offset" min=0.0 max=1.0 step=1e-05 scale=0.001..1.0 scale format="%#_2g"}
  out "Plot: All":cluster{"all rows":dbl[], "all rows":dbl[]}[](graph)
  in  "Sweep folder path":path=path "C:/data/Ultrasound/birdcage/Hg1201/Test"
  out "scan file found":bool=TRUE
  in  "source":enum16{"last scan file", "manual"}(ring)
  in  "subtract linear BG":bool
  out "complex region":T10={"max re"=1.5, "min re"=-1.5, "max im"=1.5, "min im"=-1.5, "delta re"=3.0, "delta im"=3.0, "center re"=0.0, "delta  z"=3.0+3.0i, "center im"=0.0, "center z"=0.0+0.0i, "d im"=0.0, "d re"=0.0, "d z"=0.0+0.0i}
  in  "cursor bracket: All, data window":T11={"left"=3360.8902399154335, "right "=3437.1683335733683, "center"=3399.029286744401, "window"=76.27809365793496, "cursors"=[0, 1, 2], "relative"=0, "absolute"=0, "fixed vertical offset"=0.0, "vertical offset"=0.0, "skew"=0.0, "default window frac"=0.1, "kind"=enum."symmetric", "skew.left"=0.5, "skew.right"=0.5, "Plot ref"=refnum, "wing order"=enum."forw"}
  out "all:min omega":dbl=999.9999892897904
  out "all:max omega":dbl=4999.839991796762
  in  "file path":path=path "C:/data/Ultrasound/birdcage/Hg1201/Test/September_2016/090216/300.46100K_1000_5000_2.00000V_0.00000T_Sep02-2016__15-54-27_001_090216.bin"
  in  "Tab : parameters":enum32{"Page 1"}(tab)
  out "VKey":T12
  out "Char":i16=83
  in  "parameters: complex fit":T13={"main VI path"=path "E:/ProjectLocker/LANL/Libraries/control rus sweep -- library/monitor RUS scan.vi", "scale factor"=3.0, "# of grid points"=150, "parameters: wavepacket"={"R"=0.5, "wave number"=22.0, "delta k"=7.0, "radii vector"=[], "radial section"=[], "wave vector"=22.0, "wavepacket is"=TRUE}, "span"=0.33799, "interference ?"=enum."pm zcenter", "filter method"=enum."three"} {"span" min=0.0 max=0.5 step=1e-05 scale=0.0001..0.5 scale format="%#_5f"; "parameters: wavepacket"."delta k" format="%#_3f"; "parameters: wavepacket"."wave number" format="%#_3f"; "parameters: wavepacket"."R" format="%#_3f"}
  out "4corners":T6={"z (-pi/2)"=-0.09147536254399669-0.04226381590014872i, "z(inf)"=-0.09294911564715679-0.04048496018119781i, "z (pi/2)"=-0.0947279713661077-0.041958713284357914i, "z center"=-0.09310166695505219-0.04211126459225332i, "z(0)"=-0.0932542182629476-0.04373756900330883i, "radius"=0.0016334435830353037}
  out "good lorentzian":T5={"Amplitude"=0.000340055891053764, "omega(0)"=3392.560000065714, "Gamma"=11.91999763250351, "phase"=1.0574274315248449, "Q"=284.61079478865537, "Norm  Ampl"=nan, "z (inf)"=-2.2995916620324662e-05-1.1031702558117846e-05i, "4corners"={"z (-pi/2)"=1.5865449989673634e-05-1.9155492294065609e-07i, "z(inf)"=-2.2995916620324662e-05-1.1031702558117846e-05i, "z (pi/2)"=-1.2155768985147472e-05-4.9893069168116145e-05i, "z center"=1.8548405022630806e-06-2.50423120455284e-05i, "z(0)"=2.6705597624850824e-05-3.905292153293895e-05i, "radius"=2.8528184445817156e-05}} {"z (inf)" format="%#9_9f"; "Q" format="%#9_9f"; "phase" format="%#9_9f"; "Gamma" format="%#9_9f"; "omega(0)" format="%#9_9f"}
  # "three strikes"
  # "search window"
  # "linear extrapolation"
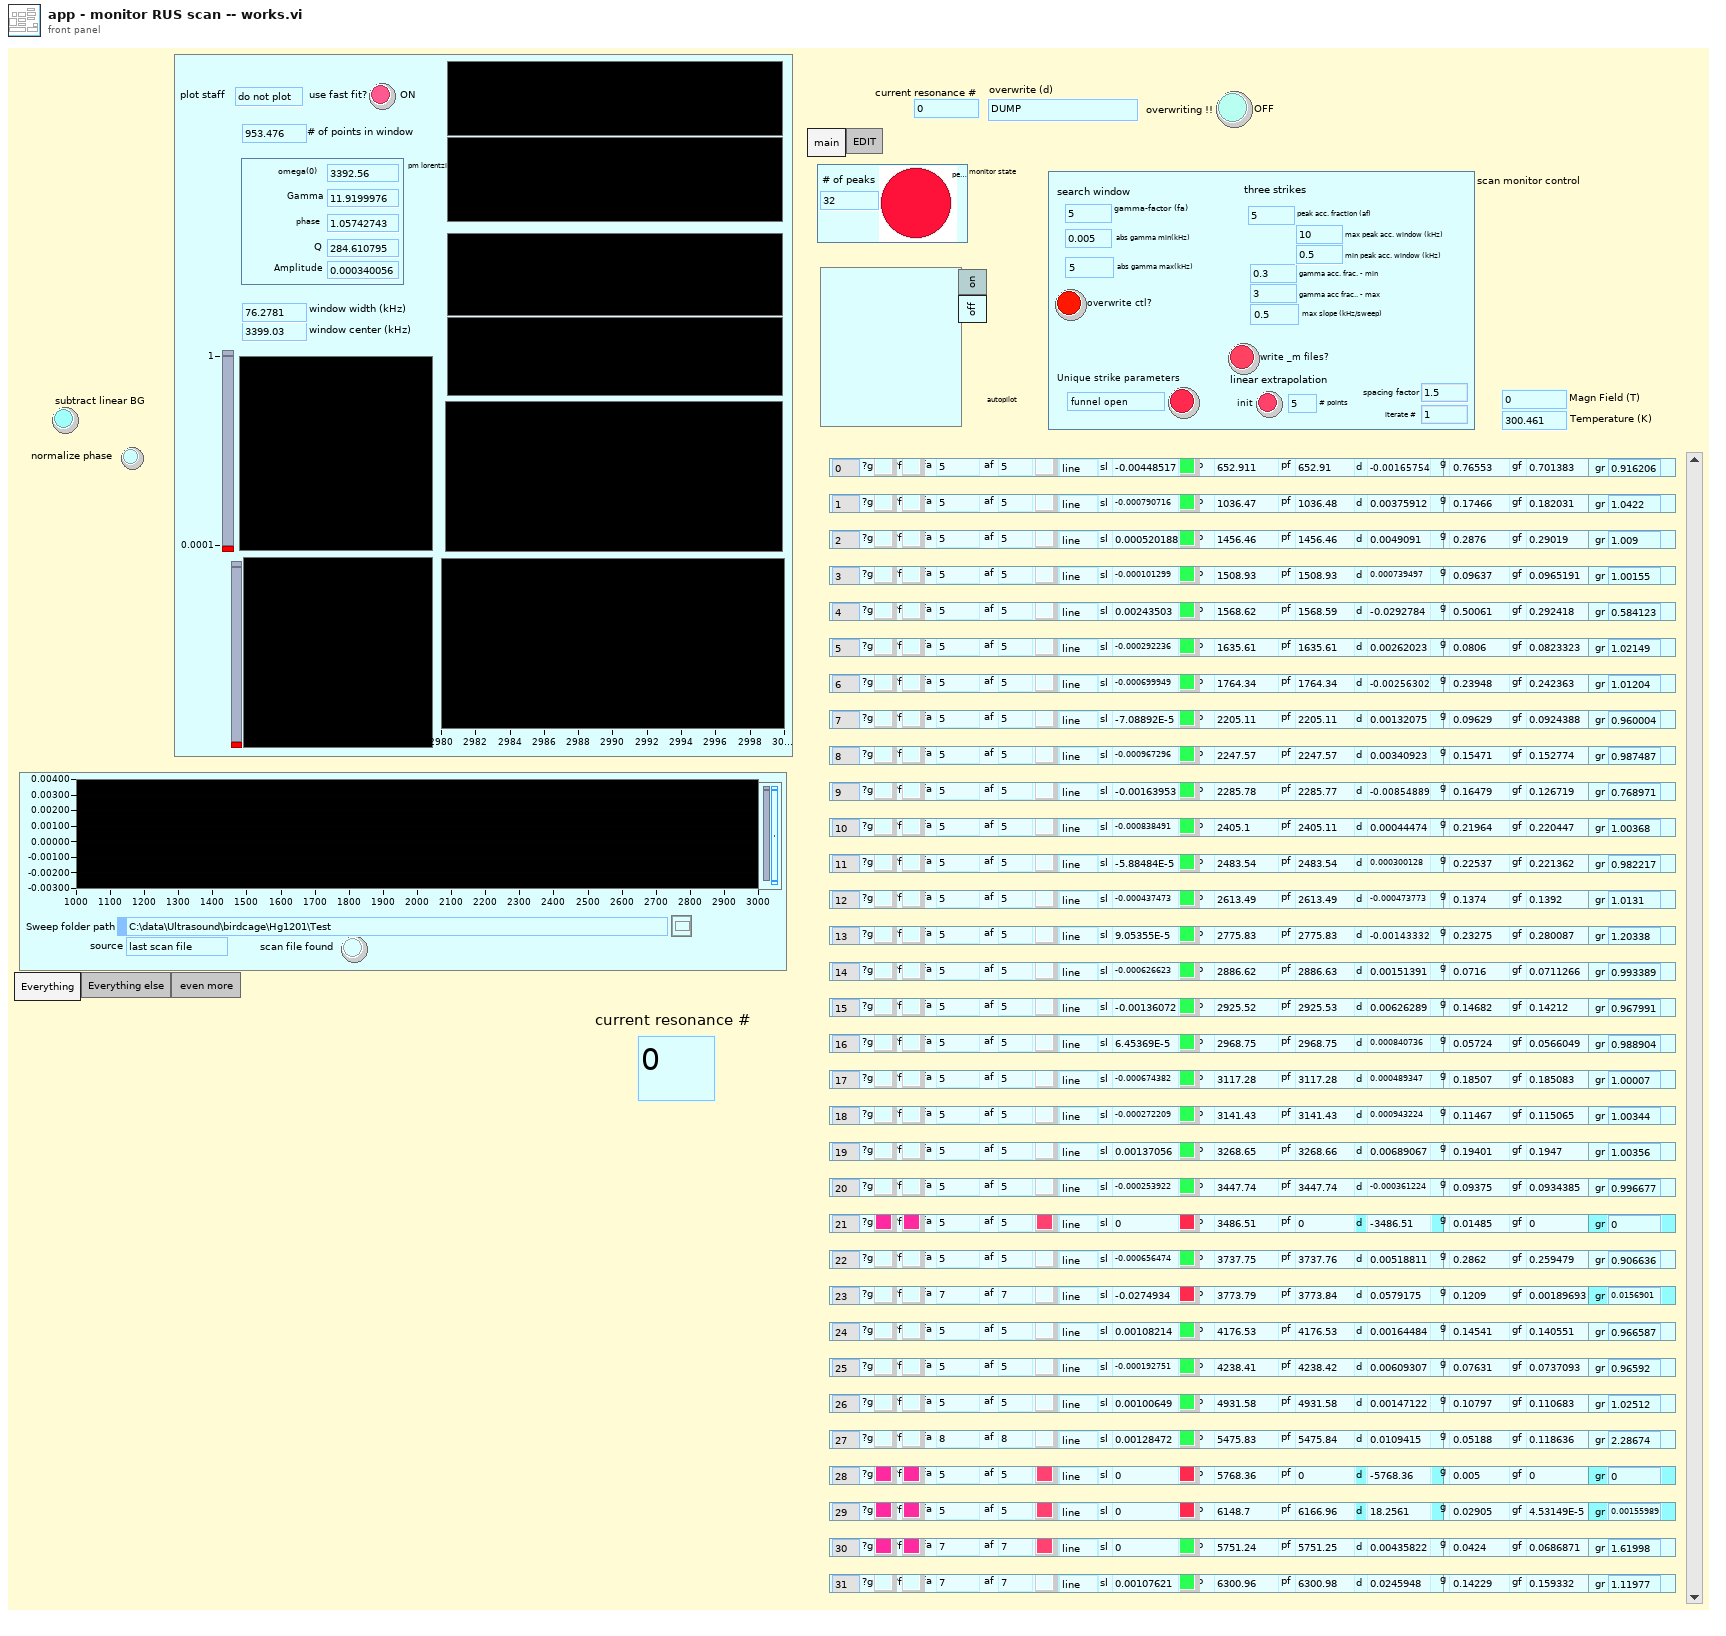
[diagram p1: front panel]
types:
  T1 = typedef "parameters -- scan monitor control.ctl" = cluster{"gamma acc. frac. - min ":dbl, "gamma acc frac.. - max":dbl, "peak acc. fraction (af)":dbl, "min peak acc. window (kHz)":dbl, "use":enum16{"window", "fraction"}, "abs gamma min(kHz)":dbl, "abs gamma max(kHz)":dbl, "# points":i32, "gamma-factor (fa)":dbl, "interpolate":enum16{"line", "last"}, "init":bool, "Unique strike parameters":bool, "max peak acc. window (kHz)":dbl, "spacing factor":dbl, "iterate #":i32, "overwrite ctl?":bool, "write _m files?":bool, "max slope (kHz/sweep)":dbl, "funnel state":enum16{"funnel open", "funnel closed"}}
  T2 = typedef "monitor state.ctl" = cluster{"header - gamma":string[], "header - frequency":string[], "# of peaks":i32, "peaks OK":bool}
  T3 = typedef "peak monitor ctl - V2.ctl" = cluster{"delta":dbl, "gamma":dbl, "exp":dbl, "found?":bool, "found":dbl, "gamma found":dbl, "init linear":bool, "interpolate":enum16{"line", "force"}, "gamma-factor":dbl, "slope":dbl, "update freq?":bool, "update gamma?":bool, "acc factor":dbl, "linear interpolation state":T4, "ind":dbl, "gamma ratio":dbl, "gamma off limit?":bool, "freq off limit?":bool}
  T4 = typedef "interpolation state - real.ctl" = cluster{"requested size":i32, "Array":dbl[], "actual number of elements":i32}
  T5 = typedef "lorentzian.ctl" = cluster{"Amplitude":dbl, "omega(0)":dbl, "Gamma":dbl, "phase":dbl, "Q":dbl, "Norm  Ampl":dbl, "z (inf)":cdb, "4corners":T6}
  T6 = typedef "circle corners.ctl" = cluster{"z (-pi/2)":cdb, "z(inf)":cdb, "z (pi/2)":cdb, "z center":cdb, "z(0)":cdb, "radius":dbl}
  T7 = enum32{"Everything", "Everything else", "even more "}
  T8 = cluster{"omega out":dbl[], "win omega out":dbl[]}
  T9 = typedef "scale - offset gauge.ctl" = cluster{"scale offset":dbl, "scale range":dbl}
  T10 = typedef "complex region.ctl" = cluster{"max re":dbl, "min re":dbl, "max im":dbl, "min im":dbl, "delta re":dbl, "delta im":dbl, "center re":dbl, "delta  z":cdb, "center im":dbl, "center z":cdb, "d im":dbl, "d re":dbl, "d z":cdb}
  T11 = typedef "cursor winow.ctl" = cluster{"left":dbl, "right ":dbl, "center":dbl, "window":dbl, "cursors":i32[], "relative":i32, "absolute":i32, "fixed vertical offset":dbl, "vertical offset":dbl, "skew":dbl, "default window frac":dbl, "kind":enum16{"symmetric", "skewed", "fancy"}, "skew.left":dbl, "skew.right":dbl, "Plot ref":refnum<vi>, "wing order":enum16{"forw", "back"}}
  T12 = typedef "eventvkey.ctl" = enum16{"ASCII", "Enter", "Return", "Shift", "Ctrl", "Alt", "Cmd", "Opt", "Caps", "NumLock", "Clear", "Break", "Up", "Down", "Left", "Right", "Insert", "Delete", "Home", "End", "PageUp", "PageDown", "Escape", "Help", "Pause", "ScrollLock", "F1", "F2", "F3", "F4", "F5", "F6", "F7", "F8", "F9", "F10", "F11", "F12", "F13", "F14", "F15", "F16", "F17", "F18", "F19", "F20", "F21", "F22", "F23", "F24", "Play", "VolumeUp", "VolumeDown", "Mute", "Two Byte Char"}
  T13 = typedef "peak -- parameters -- complex fit.ctl" = cluster{"main VI path":path, "scale factor":dbl, "# of grid points":i32, "parameters: wavepacket":T14, "span":dbl, "interference ?":enum16{"cp z center", "pm zcenter", "fancy"}, "filter method":T15}
  T14 = typedef "wavepacket.ctl" = cluster{"R":dbl, "wave number":dbl, "delta k":dbl, "radii vector":dbl[], "radial section":cdb[], "wave vector":dbl, "wavepacket is":bool}
  T15 = typedef "filter method control.ctl" = enum16{"four", "five", "one", "two", "three", "zero", "minus one", "minus two"}
  T16 = typedef "countdown control.ctl" = enum16{"check", "start", "reset cont", "stop", "reset once"}
  T17 = typedef "plot refs -- filter related.ctl" = cluster{"Plot: complex plane - filter":refnum<vi>, "Plot: dz/domega":refnum<vi>, "Plot: fragment filter":refnum<vi>, "Plot: win omega":refnum<vi>, "Plot: phase":refnum<vi>, "Plot: phase around center":refnum<vi>, "Plot: complex plane":refnum<vi>, "Plot: fragment":refnum<vi>}
  T18 = typedef "cursor window action.ctl" = enum16{"balance", "h. offset change", "cursor moves", "change center", "change window", "init", "check", "reset", "set y to middle", "idle", "-write all Y", "-write left.X", "-write center.X", "-write right.X", "-write all X", "-change center", "-change window", "-change skew", "-read cursor 2", "-read cursor 1", "-read cursor 0", "-read all cursors", "-reset", "-read plot scale", "-set y to middle", "-Q: center.Y is visible", "-Q: window is visible", "-parse center.Y", "-right left from center", "-left move", "-right move", "-set center.Y", "-empty", "-set cursors to default", "-check", "-write center.Y", "-copy cursor 1", "-copy cursor 0", "-copy cursor 2", "move right", "move left", "shrink", "broaden", "skew up", "skew down", "-write plot scale", "zoom X", "change cen&win", "zoom to all data"}
  T19 = typedef "read scan file control.ctl" = cluster{"# columns":i32, "create bin file":bool, "do not filter":bool, "normalize phase":bool, "read freq units":enum16{"kHz", "Hz"}}
  T20 = typedef "monitor action.ctl" = enum16{"monitor", "interpolate", "global", "read", "overwrite", "write m file", "nothing", "eeee"}
  T21 = typedef "ctl -- name dispatcher -- action.ctl" = enum16{"peak frequency", "peak frequency DUMP", "peak gamma DUMP", "peak gamma", "peak frequency TEST", "peak gamma TEST", "ultrasonic power", "time in gamma", "set temperature ", "set temperature timer", "peak default gamma", "last scan file", "peak freq gamma TEST", "peak NAMES", "errors", "P_I_D", "P", "I", "D", "power vs time", "power vs time TIMER", "void", "power log", "set temperature - SINE", "itc ltc log", "peak - time in gamma"}
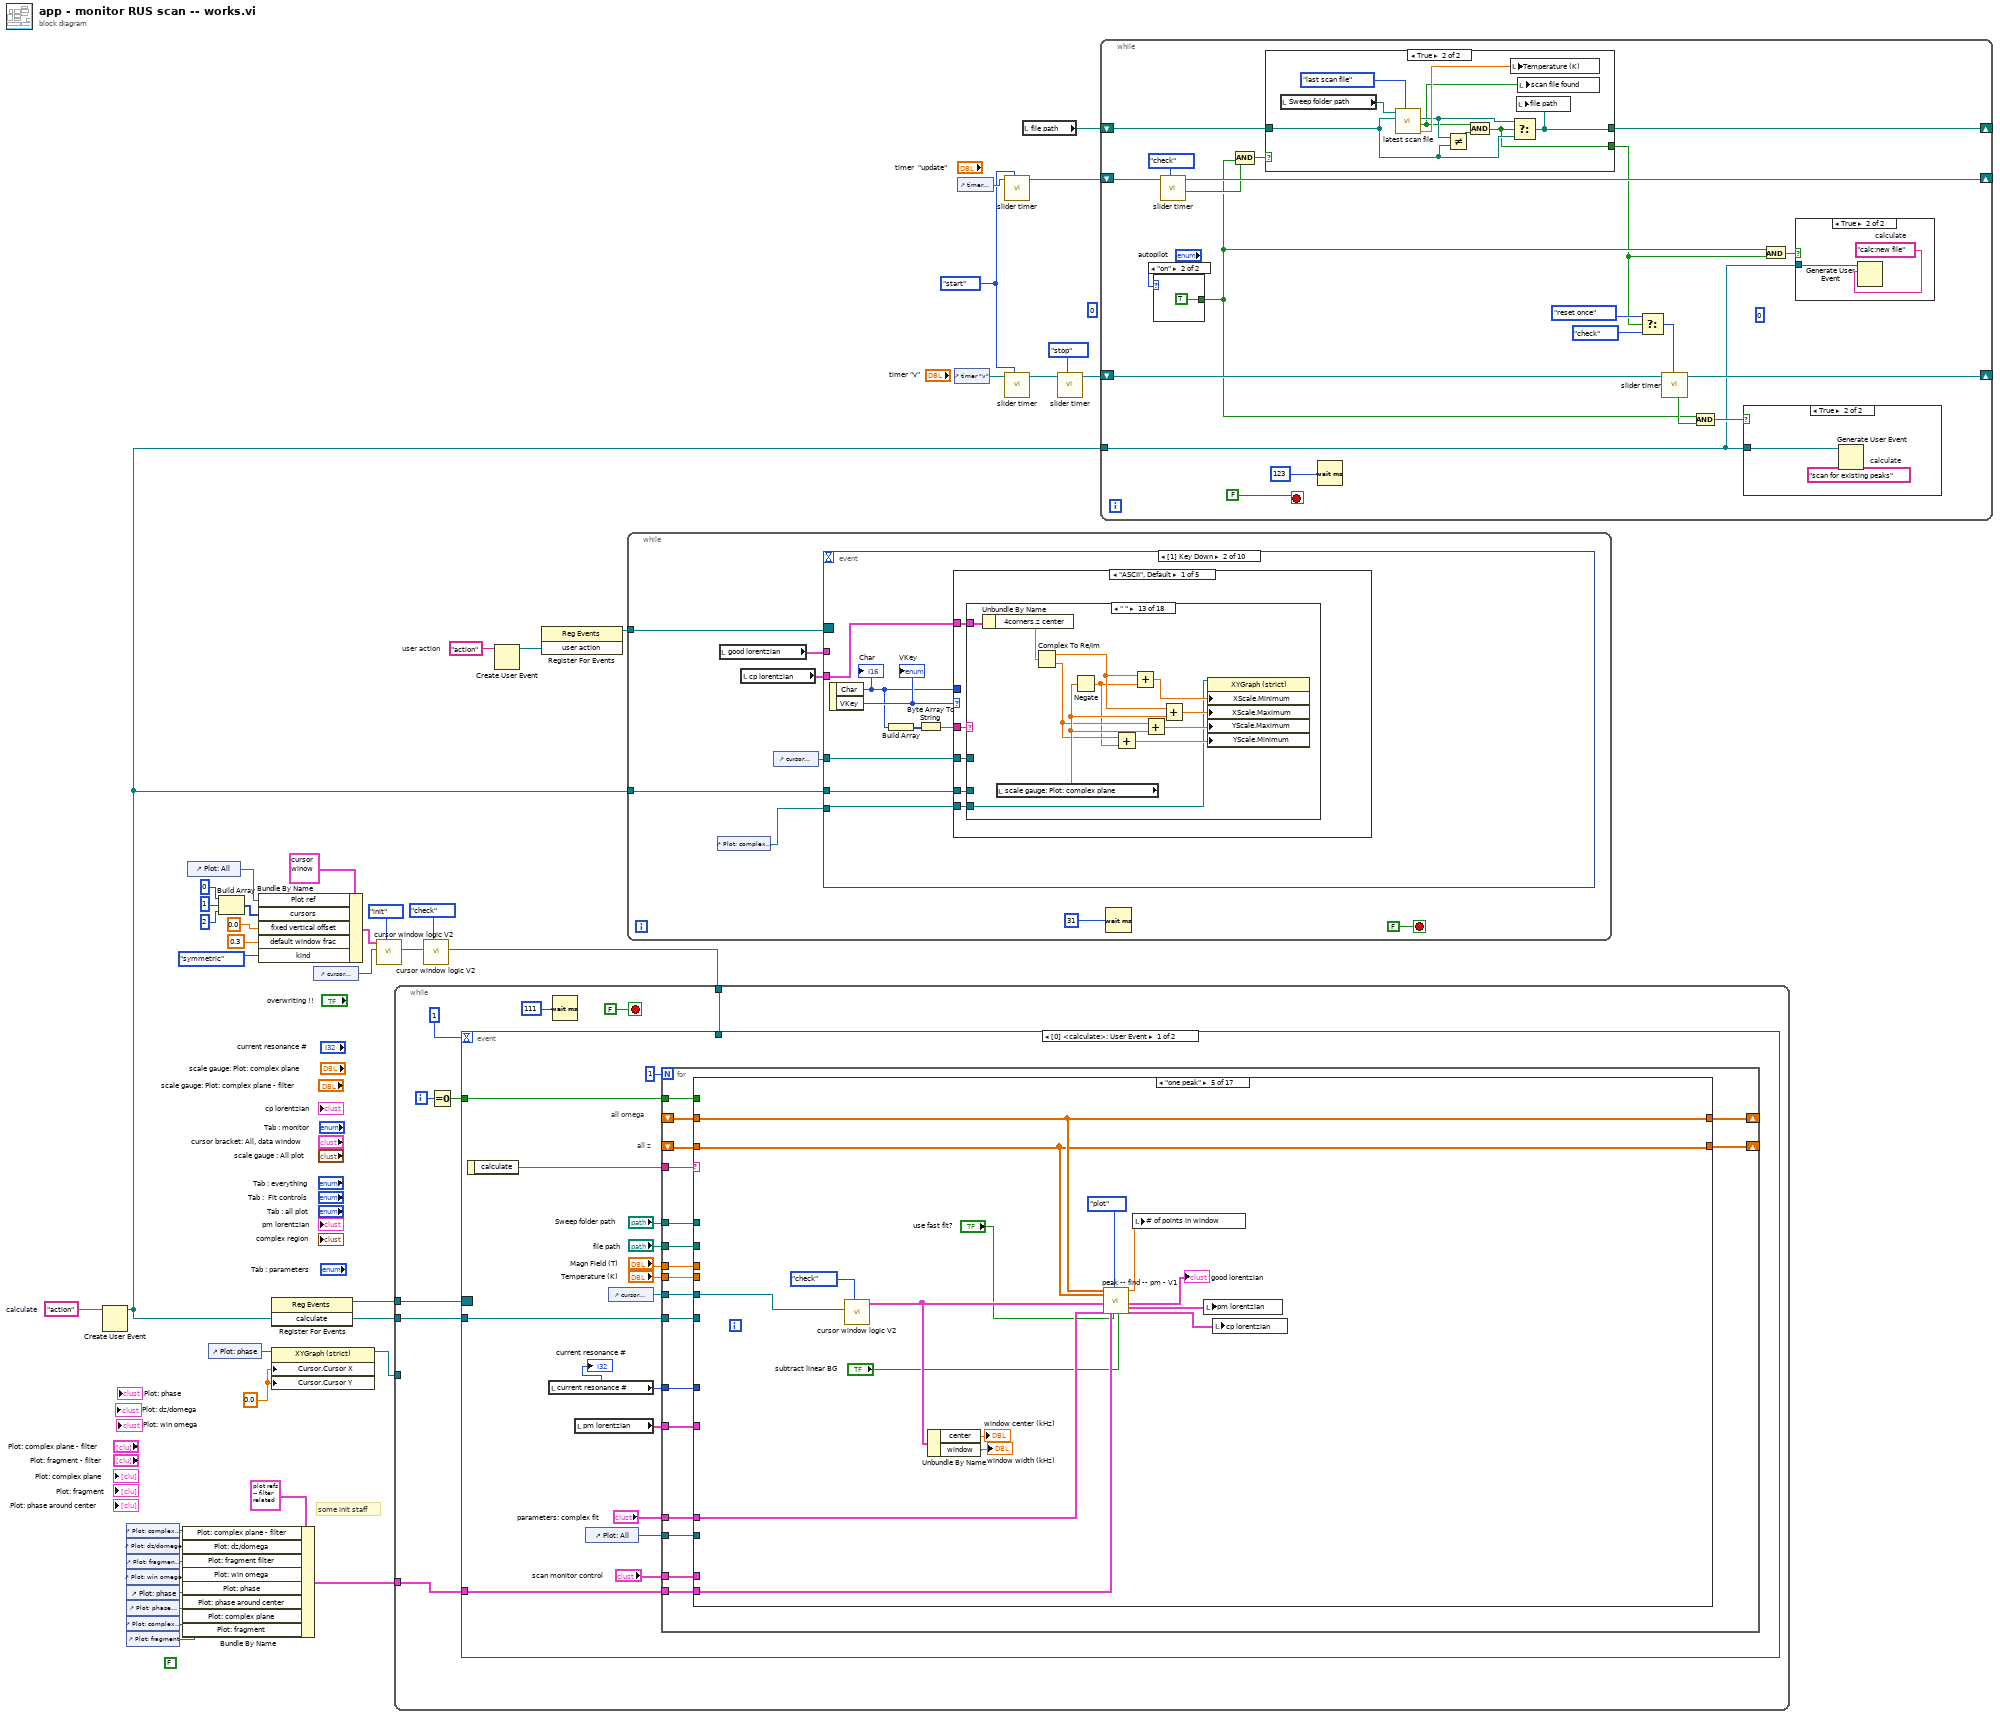
[diagram p0: block diagram]
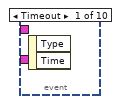
[diagram p2: hidden frame]
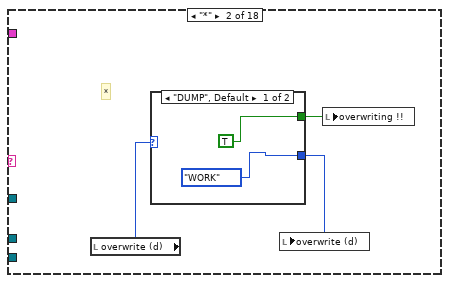
[diagram p4: hidden frame]
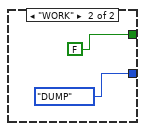
[diagram p5: hidden frame]
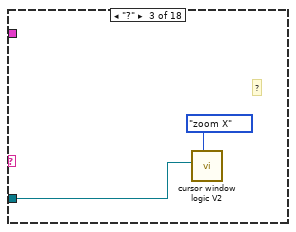
[diagram p6: hidden frame]
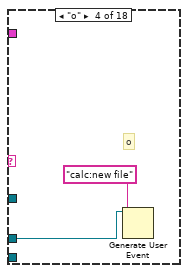
[diagram p7: hidden frame]
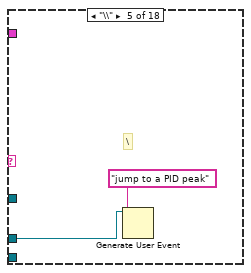
[diagram p8: hidden frame]
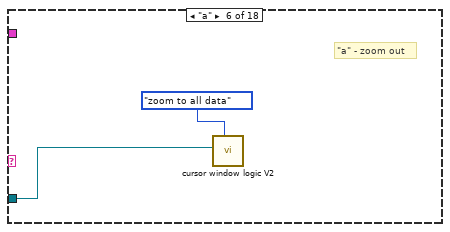
[diagram p9: hidden frame]
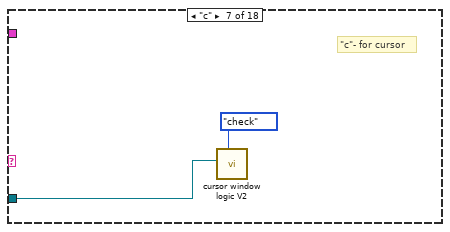
[diagram p10: hidden frame]
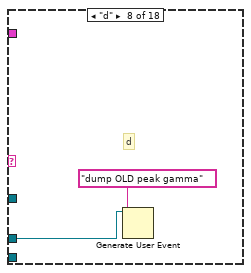
[diagram p11: hidden frame]
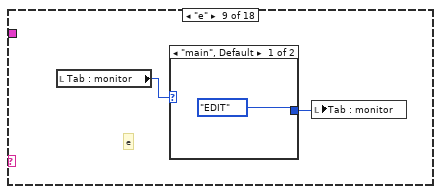
[diagram p12: hidden frame]
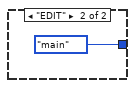
[diagram p13: hidden frame]
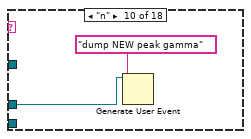
[diagram p14: hidden frame]
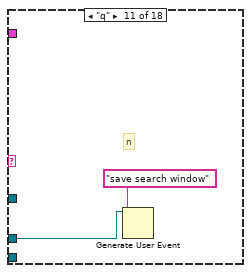
[diagram p15: hidden frame]
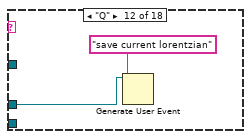
[diagram p16: hidden frame]
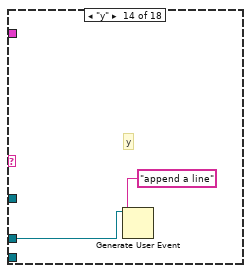
[diagram p17: hidden frame]
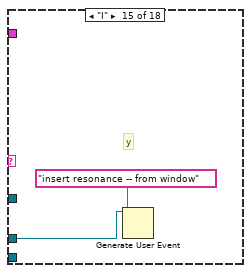
[diagram p18: hidden frame]
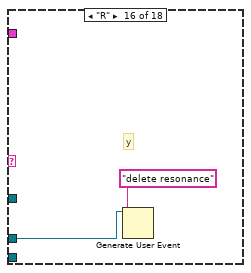
[diagram p19: hidden frame]
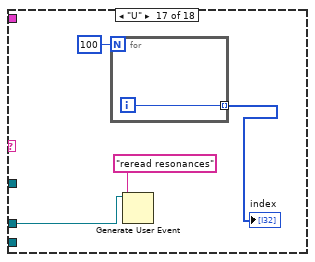
[diagram p20: hidden frame]
diagram:
  w19 = 0.0 ("Cursor.Cursor Position:Cursor X")
  w27 = "action"  # user action
  w6 = countdown_control."start" ("action")
  (unwired) 0
  w41 = "action"  # calculate
  (unwired) FALSE
  # "some init staff"
  n1 = Create User Event(user event datatype=w41) -> (user event=w25:refnum<user-event>)  [unwired: 1 in, 1 out]
  n2 = control-ref of="Plot: complex plane - filter"() -> (w16:refnum<vi>)
  n3 = control-ref of="Plot: dz/domega"() -> (w15:refnum<vi>)
  n4 = control-ref of="Plot: fragment - filter"() -> (w14:refnum<vi>)
  n5 = control-ref of="Plot: win omega"() -> (w13:refnum<vi>)
  n6 = control-ref of="Plot: phase"() -> (w12:refnum<vi>)
  n7 = control-ref of="Plot: phase around center"() -> (w10:refnum<vi>)
  n8 = control-ref of="Plot: complex plane"() -> (w9:refnum<vi>)
  n9 = control-ref of="Plot: fragment"() -> (w8:refnum<vi>)
  n10 = Bundle By Name(cluster=T17 {"Plot: complex plane - filter"=refnum, "Plot: dz/domega"=refnum, "Plot: fragment filter"=refnum, "Plot: win omega"=refnum, "Plot: phase"=refnum, "Plot: phase around center"=refnum, "Plot: complex plane"=refnum, "Plot: fragment"=refnum} ("plots: filter related"), "Plot: complex plane - filter"=w16, "Plot: dz/domega"=w15, "Plot: fragment filter"=w14, "Plot: win omega"=w13, "Plot: phase"=w12, "Plot: phase around center"=w10, "Plot: complex plane"=w9, "Plot: fragment"=w8) -> (w11:T17)
  n11 = control-ref of="Plot: All"() -> (w32:refnum<vi>)
  n12 = control-ref of="Plot: phase"() -> (w20:refnum<vi>)
  n13 = Build Array(0, 1, 2) -> (w40:i32[])
  n14 = Bundle By Name(cluster=T11 {"left"=0.0, "right "=0.0, "center"=0.0, "window"=0.0, "cursors"=[], "relative"=0, "absolute"=0, "fixed vertical offset"=0.0, "vertical offset"=0.0, "skew"=0.0, "default window frac"=0.0, "kind"=enum."symmetric", "skew.left"=0.0, "skew.right"=0.0, "Plot ref"=refnum, "wing order"=enum."forw"} ("cursor bracket: All, data window"), "Plot ref"=w32, "cursors"=w40, "fixed vertical offset"=0.0, "default window frac"=0.3 ("fixed vertical offset"), "kind"=enum16{"symmetric", "skewed", "fancy"}."symmetric") -> (w31:T11)
  n15 = register-events(w25) -> (reference out=w42:refnum<event-registration>)  [unwired: 2 in, 1 out]
  n16 = property class="XYGraph (strict)"(reference=w20, "Cursor.Cursor X"=w19, "Cursor.Cursor Y"=w19) -> (reference out=w18:refnum<vi>)  [unwired: 1 in, 1 out]
  n17 = control-ref of="cursor bracket: All, data window"() -> (w30:refnum<vi>)
  n18 = call "cursor window logic V2.vi"("cursor window action"=cursor_window_action."init", "cursor window in"=w30, "cursor window init"=w31) -> ("cursor window out"=w23:refnum<vi>)  [unwired: 7 in, 1 out]
  n19 = call "cursor window logic V2.vi"("cursor window action"=cursor_window_action."check", "cursor window in"=w23) -> ("cursor window out"=w21:refnum<vi>)  [unwired: 8 in, 1 out]
  n20 = while {
    tunnel: w42 -> [w51]
    tunnel: w25 -> [w49]
    tunnel: w21 -> [w45]
    tunnel: w18 -> [_]
    tunnel: w11 -> [w44]
    i -> [w46]
    stop <- FALSE stop-if-true
    n21 = Equal To 0?(x=w46) -> (x = 0?=w43:bool)
    n22 = event shown="[0] <calculate>: User Event" {
      selector: w51 -> [_ _]
      dyn-events: _ -> [_ _]
      timeout: 1 -> [_ _]
      tunnel: w49 -> [w65 _]
      tunnel: w45 -> [_ _]
      tunnel: w44 -> [w60 _]
      tunnel: w43 -> [w59 _]
      event User Event {
        # "all z"
        # "all omega"
        n23 = event-data() -> ("calculate"=w66:string)  [unwired: 1 in]
        n24 = local read "current resonance #"() -> (w52:i32)
        "current resonance #" <- w52
        n25 = local read "pm lorentzian"() -> (w53:T5)
        n26 = control-ref of="Plot: All"() -> (w63:refnum<vi>)
        n27 = control-ref of="cursor bracket: All, data window"() -> (w54:refnum<vi>)
        n28 = for {
          N: 1 -> [_]
          tunnel: w66 -> [w84]
          tunnel: w65 -> [w83]
          shift-right: [w80] -> _
          shift-left: _ -> [w82]
          shift-right: [w79] -> _
          shift-left: _ -> [w81]
          tunnel: w54 -> [w78]
          tunnel: w63 -> [w77]
          tunnel: "Sweep folder path" -> [w76]
          tunnel: "Temperature (K)" -> [w75]
          tunnel: w52 -> [w74]
          tunnel: w60 -> [w73]
          tunnel: w59 -> [w72]
          tunnel: "parameters: complex fit" -> [w71]
          tunnel: "file path" -> [w70]
          tunnel: "scan monitor control" -> [w69]
          tunnel: "Magn Field (T)" -> [w68]
          tunnel: w53 -> [w67]
          n29 = case shown="\"one peak\"" w84 {
            tunnel: w83 -> [_ _ _ _ _ _ _ _ _ _ _ w310 w328 w343 w357 _ _]
            tunnel: w82 -> [w91 w149 w197 w212 w241 w246 w258 w274 w285 w294 w296 w309 w327 w342 w356 w370 w379]
            tunnel: w81 -> [w90 w148 w196 w211 w240 w245 w257 w273 w284 w293 w295 w308 w326 w341 w355 w369 w378]
            tunnel: [w95 w149 w197 w212 w241 w246 w258 w274 w285 w294 w296 w309 w327 w342 w356 w370 w379] -> w80
            tunnel: [w94 w148 w196 w211 w240 w245 w257 w273 w284 w293 w295 w308 w326 w341 w355 w369 w378] -> w79
            tunnel: w78 -> [_ w147 _ _ w242 _ _ _ _ _ _ w311 w329 w344 w358 _ _]
            tunnel: w77 -> [_ _ _ _ _ _ _ _ _ _ _ _ _ _ _ _ _]
            tunnel: w76 -> [w93 w117 w193 w210 _ _ _ _ _ _ _ _ _ _ _ w363 w398]
            tunnel: w75 -> [_ w116 w189 w209 _ _ _ _ _ _ _ _ _ _ _ w361 _]
            tunnel: w74 -> [_ _ _ _ _ w244 w255 w267 w276 w287 _ w307 w325 w340 w346 _ _]
            tunnel: w73 -> [_ w146 _ _ w235 _ _ _ _ _ _ _ _ _ _ _ _]
            tunnel: w72 -> [_ w138 _ _ _ _ _ _ _ _ _ _ _ _ _ _ _]
            tunnel: w71 -> [_ w145 _ _ w234 _ _ _ _ _ _ _ _ _ _ _ _]
            tunnel: w70 -> [w87 _ _ _ _ _ _ _ _ _ _ _ _ _ _ _ _]
            tunnel: w69 -> [_ w114 _ _ _ _ _ _ _ _ _ _ _ _ _ _ _]
            tunnel: w68 -> [_ w113 _ _ _ _ _ _ _ _ _ _ _ _ _ _ _]
            tunnel: w67 -> [_ _ _ _ _ _ w256 w272 w283 w292 _ _ _ _ _ _ _]
            frame "calc:new file" {
              n30 = call "latest scan file.vi"("source"="source", "file path in"=w87, "sweep folder"=w93) -> ("temperature (K)"=w89:dbl, "file or folder exists?"=w92:bool, "file path out"=w88:path, "Magn Field (T)"=w85:dbl)  [unwired: 5 in]
              "scan file found" <- w92
              n31 = case shown="True" w92 {
                tunnel: [w97 w110] -> w95
                tunnel: [w96 w109] -> w94
                tunnel: w88 -> [_ w108]
                tunnel: w91 -> [w97 _]
                tunnel: w90 -> [w96 _]
                frame False {
                }
                frame True {
                  # "Hz/kHz"
                  n32 = Bundle By Name(cluster=T19 {"# columns"=3, "create bin file"=TRUE, "do not filter"=TRUE, "normalize phase"=FALSE, "read freq units"=enum."kHz"} ("read scan file"), "normalize phase"="normalize phase") -> (w99:T19)
                  n33 = call "rus fit - load data file.vi"("file path"=w108, "read scan file"=w99) -> ("all:max omega"=→"all:max omega":dbl, "all:min omega"=→"all:min omega":dbl, "omega"=w110:dbl[], "x + iy"=w109:cdb[])  [unwired: 5 in, 1 out]
                  n34 = Complex To Re/Im(x + iy=w109) -> (x=w102:dbl[], y=w101:dbl[])
                  n35 = Bundle("omega"=w110, w102) -> (w103:cluster{"omega":dbl[], dbl[]})  [unwired: 1 in]
                  n36 = Bundle("omega"=w110, w101) -> (w104:cluster{"omega":dbl[], dbl[]})  [unwired: 1 in]
                  n37 = Build Array(w103, w104) -> (→"Plot: All":cluster{"omega":dbl[], dbl[]}[])
                }
              }
              n38 = local write "file path"(w88) -> ()
              n39 = local write "Magn Field (T)"(w85) -> ()
              n40 = local write "Temperature (K)"(w89) -> ()
            }
            frame "scan for existing peaks" {
              (unwired) 0 ("length")
              (unwired) 1.0 ("element")
              n41 = local read "Array of states"() -> (w144:T3[])
              n42 = local read "monitor state"() -> (w126:T2)
              n43 = Unbundle By Name(w114) -> ("iterate #"=w139:i32)
              n44 = call "monitor scan logic.vi"("Array IN"=w144, "monitor action"=monitor_action."read", "monitor state"=w126, "scan monitor control IN"=w114, "Sweep folder path"=w117, "temperature"=w116) -> ("Array OUT"=w129:T3[], "freq OUT"=w127:dbl[], "gamma OUT"=w128:dbl[], "monitor state OUT"=w134:T2)  [unwired: 6 in]
              n45 = call "monitor scan logic.vi"("Array IN"=w129, "monitor action"=monitor_action."global", "freq IN"=w127, "gamma IN"=w128, "monitor state"=w134, "scan monitor control IN"=w114) -> ("Array OUT"=w137:T3[], "freq OUT"=w136:dbl[], "gamma OUT"=w135:dbl[], "monitor state OUT"=w133:T2)  [unwired: 6 in]
              n46 = for {
                N: w139 -> [_]
                tunnel: w149 -> [w165]
                tunnel: w148 -> [w164]
                tunnel: w147 -> [w163]
                tunnel: w146 -> [w158]
                tunnel: w145 -> [w157]
                tunnel: w114 -> [w156]
                shift-right: [w154] -> w142
                shift-left: w136 -> [w161]
                shift-right: [w160] -> w141
                shift-left: w135 -> [w155]
                shift-right: [w159] -> w140
                shift-left: w137 -> [w153]
                shift-right: [w152] -> w132
                shift-left: w133 -> [w152]
                tunnel: "plot staff" -> [w151]
                tunnel: monitor_action."monitor" ("monitor action") -> [w150]
                n47 = for {
                  tunnel: w161 -> [w182] mode=indexing
                  tunnel: w163 -> [w185]
                  tunnel: w165 -> [w177]
                  tunnel: w164 -> [w176]
                  tunnel: [w183] -> w162 mode=indexing
                  tunnel: w155 -> [w179] mode=indexing
                  tunnel: w158 -> [w174]
                  tunnel: w157 -> [w173]
                  tunnel: w153 -> [w169] mode=indexing
                  tunnel: w151 -> [w167]
                  n48 = Unbundle By Name(w169) -> ("gamma-factor"=w168:dbl)
                  n49 = Multiply(x=w168, y=w179) -> (x*y=w181:dbl)
                  n50 = call "cursor window logic V2.vi"("cursor window action"=cursor_window_action."change cen&win", "window"=w181, "center"=w182, "cursor window in"=w185) -> ("cursor window out"=w170:T11)  [unwired: 6 in, 1 out]
                  n51 = call "peak -- find -- pm - V1.vi"("omega in"=w177, "z in"=w176, "cursor window"=w170, "parameters: complex fit"=w173, "plots: filter related"=w174, "plot staff ?"=w167) -> ("# points in window"=→"# of points in window":dbl, "good lorentzian"=w171:T5, "pm lorentzian"=w178:T5, "cp lorentzian"=w172:T5)  [unwired: 10 in]
                  n52 = Unbundle By Name(w171) -> ("omega(0)"=w175:dbl, "Gamma"=w180:dbl)
                  n53 = local write "pm lorentzian"(w178) -> ()
                  n54 = local write "cp lorentzian"(w172) -> ()
                  n55 = Bundle By Name(cluster=w169, "exp"=w182, "found"=w175, "gamma"=w179, "gamma found"=w180) -> (w183:T3)
                }
                n56 = call "monitor scan logic.vi"("Array IN"=w162, "monitor action"=w150, "scan monitor control IN"=w156) -> ("Array OUT"=w159:T3[], "freq OUT"=w154:dbl[], "gamma OUT"=w160:dbl[])  [unwired: 9 in, 1 out]
              }
              n57 = local write "OLD gamma"(w128) -> ()
              n58 = local write "OLD freq"(w127) -> ()
              n59 = call "monitor scan logic.vi"("Array IN"=w140, "monitor action"=monitor_action."interpolate", "init"=w138, "freq IN"=w142, "gamma IN"=w141, "monitor state"=w132, "scan monitor control IN"=w114) -> ("Array OUT"=w125:T3[], "freq OUT"=w123:dbl[], "gamma OUT"=w122:dbl[], "monitor state OUT"=w121:T2)  [unwired: 5 in]
              n60 = call "monitor scan logic.vi"("Array IN"=w125, "monitor action"=monitor_action."overwrite", "freq IN"=w123, "Magn Field (T)"=w113, "gamma IN"=w122, "monitor state"=w121, "scan monitor control IN"=w114, "Sweep folder path"=w117, "temperature"=w116) -> ("Array OUT"=w124:T3[], "freq OUT"=w118:dbl[], "gamma OUT"=w119:dbl[], "monitor state OUT"=w120:T2)  [unwired: 3 in]
              n61 = local write "Array of states"(w124) -> ()
              n62 = local write "NEW freq"(w118) -> ()
              n63 = local write "NEW gamma"(w119) -> ()
              n64 = local write "monitor state"(w120) -> ()
            }
            frame "dump OLD peak gamma" {
              w192 = enum16{"append", "overwrite"}."overwrite" ("append/overwrite")
              n65 = local read "OLD gamma"() -> (w190:dbl[])
              n66 = local read "OLD freq"() -> (w194:dbl[])
              n67 = case shown="\"WORK\"" "overwrite (d)" {
                tunnel: [ctl_--_name_dispatcher_--_action."peak frequency DUMP" ("ctl name dispatch") ctl_--_name_dispatcher_--_action."peak frequency" ("ctl name dispatch")] -> w195
                tunnel: [ctl_--_name_dispatcher_--_action."peak gamma DUMP" ("ctl name dispatch") ctl_--_name_dispatcher_--_action."peak gamma" ("ctl name dispatch")] -> w191
                tunnel: [enum16{"DUMP", "WORK", ""}."DUMP" ("dump/work") enum16{"DUMP", "WORK", ""}."DUMP" ("dump/work")] -> w187
                tunnel: [FALSE ("overwriting !!") FALSE ("overwriting !!")] -> w186
                frame "DUMP", Default {
                }
                frame "WORK" {
                }
              }
              n68 = call "PID append overwrite.vi"("temperature"=w189, "append/overwrite"=w192, "PID freq"=w194, "ctl kind IN"=w195, "sweep folder"=w193) -> ()  [unwired: 6 in, 1 out]
              n69 = call "PID append overwrite.vi"("temperature"=w189, "append/overwrite"=w192, "PID freq"=w190, "ctl kind IN"=w191, "sweep folder"=w193) -> ()  [unwired: 6 in, 1 out]
              n70 = local write "overwriting !!"(w186) -> ()
              n71 = local write "overwrite (d)"(w187) -> ()
            }
            frame "dump NEW peak gamma" {
              n72 = case shown="True" TRUE {
                tunnel: w210 -> [_ w221]
                tunnel: w209 -> [_ w220]
                frame False {
                }
                frame True {
                  w217 = enum16{"append", "overwrite"}."overwrite" ("append/overwrite")
                  n73 = local read "NEW gamma"() -> (w215:dbl[])
                  n74 = local read "NEW freq"() -> (w218:dbl[])
                  n75 = case shown="\"DUMP\", Default" "dump/work NEW (\"n\")" {
                    tunnel: [ctl_--_name_dispatcher_--_action."peak frequency DUMP" ("ctl name dispatch") ctl_--_name_dispatcher_--_action."peak frequency" ("ctl name dispatch")] -> w219
                    tunnel: [ctl_--_name_dispatcher_--_action."peak gamma DUMP" ("ctl name dispatch") ctl_--_name_dispatcher_--_action."peak gamma" ("ctl name dispatch")] -> w216
                    tunnel: [enum16{"DUMP", "WORK", ""}."DUMP" ("dump/work") enum16{"DUMP", "WORK", ""}."DUMP" ("dump/work")] -> w213
                    frame "DUMP", Default {
                    }
                    frame "WORK" {
                    }
                  }
                  n76 = call "PID append overwrite.vi"("temperature"=w220, "append/overwrite"=w217, "PID freq"=w218, "ctl kind IN"=w219, "sweep folder"=w221) -> ()  [unwired: 6 in, 1 out]
                  n77 = local write "dump/work NEW (\"n\")"(w213) -> ()
                  n78 = call "PID append overwrite.vi"("temperature"=w220, "append/overwrite"=w217, "PID freq"=w215, "ctl kind IN"=w216, "sweep folder"=w221) -> ()  [unwired: 6 in, 1 out]
                }
              }
              n79 = local read "NEW gamma"() -> (w208:dbl[])
              n80 = local read "NEW freq"() -> (w207:dbl[])
              n81 = local write "OLD gamma"(w208) -> ()
              n82 = local write "OLD freq"(w207) -> ()
            }
            frame "one peak" {
              n83 = call "cursor window logic V2.vi"("cursor window action"=cursor_window_action."check", "cursor window in"=w242) -> ("cursor window out"=w239:T11)  [unwired: 8 in, 1 out]
              n84 = Unbundle By Name(w239) -> ("center"=→"window center (kHz)":dbl, "window"=→"window width (kHz)":dbl)
              n85 = call "peak -- find -- pm - V1.vi"("omega in"=w241, "z in"=w240, "cursor window"=w239, "parameters: complex fit"=w234, "plots: filter related"=w235, "plot staff ?"=enum16{"plot", "do not plot", "a"}."plot", "just guess?"="use fast fit?", "subtract linear BG"="subtract linear BG") -> ("# points in window"=w232:dbl, "good lorentzian"=→"good lorentzian":T5, "pm lorentzian"=w236:T5, "cp lorentzian"=w233:T5)  [unwired: 8 in]
              n86 = local write "# of points in window"(w232) -> ()
              n87 = local write "pm lorentzian"(w236) -> ()
              n88 = local write "cp lorentzian"(w233) -> ()
            }
            frame "save search window" {
              n89 = local read "OLD gamma"() -> (w249:dbl[])
              n90 = local read "OLD freq"() -> (w250:dbl[])
              n91 = in-place {
                n92 = in-place-array #1(w250, w244) -> ()  [unwired: 1 out]
                n93 = local read "window center (kHz)"() -> (w252:dbl)
                n94 = in-place-array #1(w252) -> (w247:dbl[])  [unwired: 1 out]
              }
              n95 = in-place {
                n96 = in-place-array #2(w249, w244) -> ()  [unwired: 1 out]
                n97 = local read "window width (kHz)"() -> (w251:dbl)
                n98 = in-place-array #2(w251) -> (w248:dbl[])  [unwired: 1 out]
              }
              n99 = local write "OLD freq"(w247) -> ()
              n100 = local write "OLD gamma"(w248) -> ()
            }
            frame "save current lorentzian" {
              n101 = local read "OLD gamma"() -> (w261:dbl[])
              n102 = local read "OLD freq"() -> (w262:dbl[])
              n103 = Unbundle By Name(w256) -> ("omega(0)"=w254:dbl, "Gamma"=w253:dbl)
              n104 = in-place {
                in-place-border: w254 -> [w264]
                n105 = in-place-array #3(w262, w255) -> ()  [unwired: 1 out]
                n106 = in-place-array #3(w264) -> (w259:dbl[])  [unwired: 1 out]
              }
              n107 = in-place {
                in-place-border: w253 -> [w263]
                n108 = in-place-array #4(w261, w255) -> ()  [unwired: 1 out]
                n109 = in-place-array #4(w263) -> (w260:dbl[])  [unwired: 1 out]
              }
              n110 = local write "OLD freq"(w259) -> ()
              n111 = local write "OLD gamma"(w260) -> ()
            }
            frame "insert resonance -- from lorentzian" {
              n112 = local read "OLD gamma"() -> (w269:dbl[])
              n113 = local read "OLD freq"() -> (w271:dbl[])
              n114 = Unbundle By Name(w272) -> ("omega(0)"=w266:dbl, "Gamma"=w265:dbl)
              n115 = Insert Into Array(array=w271, index=w267, new element=w266) -> (w270:dbl[])
              n116 = Insert Into Array(array=w269, index=w267, new element=w265) -> (w268:dbl[])
              n117 = local write "OLD freq"(w270) -> ()
              n118 = local write "OLD gamma"(w268) -> ()
            }
            frame "insert resonance -- from window" {
              n119 = local read "window center (kHz)"() -> (w281:dbl)
              n120 = local read "window width (kHz)"() -> (w277:dbl)
              n121 = local read "OLD gamma"() -> (w279:dbl[])
              n122 = local read "OLD freq"() -> (w282:dbl[])
              n123 = Unbundle By Name(w283) -> ()  [unwired: 2 out]
              n124 = call "array -- incert after.vi"("index"=w276, "Array"=w282, "number"=w281) -> ("array out"=w280:dbl[])  [unwired: 7 in, 1 out]
              n125 = call "array -- incert after.vi"("index"=w276, "Array"=w279, "number"=w277) -> ("array out"=w278:dbl[], "new index"=w275:i32)  [unwired: 7 in]
              n126 = local write "OLD freq"(w280) -> ()
              n127 = local write "OLD gamma"(w278) -> ()
              n128 = local write "current resonance #"(w275) -> ()
            }
            frame "delete resonance" {
              w286 = 1 ("length")
              n129 = local read "OLD gamma"() -> (w289:dbl[])
              n130 = local read "OLD freq"() -> (w291:dbl[])
              n131 = Unbundle By Name(w292) -> ()  [unwired: 2 out]
              n132 = Delete From Array(array=w291, length=w286, index=w287) -> (array with subset deleted=w290:dbl[])  [unwired: 1 out]
              n133 = Delete From Array(array=w289, length=w286, index=w287) -> (array with subset deleted=w288:dbl[])  [unwired: 1 out]
              n134 = local write "OLD freq"(w290) -> ()
              n135 = local write "OLD gamma"(w288) -> ()
            }
            frame "aaa", Default {
            }
            frame "jump to a PID peak" {
              w298 = "one peak"  # event data
              n136 = local read "OLD freq"() -> (w312:dbl[])
              n137 = case shown="True" TRUE {
                tunnel: w307 -> [w313 w315]
                tunnel: [w313 w314] -> w306
                frame False {
                }
                frame True {
                  n138 = Increment(x=w315) -> (x+1=w314:i32)
                }
              }
              n139 = Generate User Event(user event=w310, event data cluster=w298) -> ()  [unwired: 2 in, 2 out]
              n140 = Array Size(array=w312) -> (size(s)=w303:i32)
              n141 = Equal To 0?(x=w303) -> (x = 0?=w305:bool)
              n142 = Select(t=1, s=w305, f=w303) -> (s? t:f=w302:i32)
              n143 = Quotient & Remainder(x=w306, y=w302) -> (x-y*floor(x/y)=w299:i32)  [unwired: 1 out]
              n144 = local write "current resonance #"(w299) -> ()
              n145 = Index Array(array=w312, index=w299) -> (element=w300:dbl)
              n146 = call "cursor window logic V2.vi"("cursor window action"=cursor_window_action."change center", "center"=w300, "cursor window in"=w311) -> ()  [unwired: 7 in, 2 out]
            }
            frame "next resonance" {
              (unwired) TRUE
              w316 = "one peak"  # event data
              n147 = local read "OLD freq"() -> (w330:dbl[])
              n148 = Generate User Event(user event=w328, event data cluster=w316) -> ()  [unwired: 2 in, 2 out]
              n149 = Increment(x=w325) -> (x+1=w324:i32)
              n150 = Array Size(array=w330) -> (size(s)=w321:i32)
              n151 = Equal To 0?(x=w321) -> (x = 0?=w323:bool)
              n152 = Select(t=1, s=w323, f=w321) -> (s? t:f=w320:i32)
              n153 = Quotient & Remainder(x=w324, y=w320) -> (x-y*floor(x/y)=w317:i32)  [unwired: 1 out]
              n154 = local write "current resonance #"(w317) -> ()
              n155 = Index Array(array=w330, index=w317) -> (element=w318:dbl)
              n156 = call "cursor window logic V2.vi"("cursor window action"=cursor_window_action."change center", "center"=w318, "cursor window in"=w329) -> ()  [unwired: 7 in, 2 out]
            }
            frame "prev resonance" {
              (unwired) TRUE
              w331 = "one peak"  # event data
              n157 = local read "OLD freq"() -> (w345:dbl[])
              n158 = Generate User Event(user event=w343, event data cluster=w331) -> ()  [unwired: 2 in, 2 out]
              n159 = Decrement(x=w340) -> (x-1=w339:i32)
              n160 = Array Size(array=w345) -> (size(s)=w336:i32)
              n161 = Equal To 0?(x=w336) -> (x = 0?=w338:bool)
              n162 = Select(t=1, s=w338, f=w336) -> (s? t:f=w335:i32)
              n163 = Quotient & Remainder(x=w339, y=w335) -> (x-y*floor(x/y)=w332:i32)  [unwired: 1 out]
              n164 = local write "current resonance #"(w332) -> ()
              n165 = Index Array(array=w345, index=w332) -> (element=w333:dbl)
              n166 = call "cursor window logic V2.vi"("cursor window action"=cursor_window_action."change center", "center"=w333, "cursor window in"=w344) -> ()  [unwired: 7 in, 2 out]
            }
            frame "jump to a resonance" {
              (unwired) TRUE
              w347 = "one peak"  # event data
              n167 = local read "OLD freq"() -> (w359:dbl[])
              n168 = Generate User Event(user event=w357, event data cluster=w347) -> ()  [unwired: 2 in, 2 out]
              n169 = Array Size(array=w359) -> (size(s)=w352:i32)
              n170 = Equal To 0?(x=w352) -> (x = 0?=w354:bool)
              n171 = Select(t=1, s=w354, f=w352) -> (s? t:f=w351:i32)
              n172 = Quotient & Remainder(x=w346, y=w351) -> (x-y*floor(x/y)=w348:i32)  [unwired: 1 out]
              n173 = local write "current resonance #"(w348) -> ()
              n174 = Index Array(array=w359, index=w348) -> (element=w349:dbl)
              n175 = call "cursor window logic V2.vi"("cursor window action"=cursor_window_action."change center", "center"=w349, "cursor window in"=w358) -> ()  [unwired: 7 in, 2 out]
            }
            frame "reread resonances" {
              (unwired) TRUE
              n176 = call "PID -- read interpolate.vi"("sweep folder path"=w363, "ctl PID file IN"=ctl_--_name_dispatcher_--_action."peak frequency" ("ctl name dispatch"), "temperature"=w361) -> ("sweep folder path out"=w367:path, "PID freq"=w362:dbl[], "length out"=w364:i32)  [unwired: 11 in, 3 out]
              n177 = call "PID -- read interpolate.vi"("sweep folder path"=w367, "ctl PID file IN"=ctl_--_name_dispatcher_--_action."peak gamma" ("ctl name dispatch"), "length"=w364, "default"=1.0 ("element")) -> ("PID freq"=w360:dbl[])  [unwired: 10 in, 5 out]
              n178 = local write "OLD gamma"(w360) -> ()
              n179 = local write "OLD freq"(w362) -> ()
            }
            frame "append a line" {
              (unwired) "ctl_PID_peak_gamma_NEW.dat" ("freq PID file IN")
              w400 = 0.0 ("lower")
              n180 = call "ctl -- name dispatcher.vi"("ctl name dispatch"=ctl_--_name_dispatcher_--_action."peak frequency TEST") -> ("ctl file name"=w375:string)  [unwired: 8 in, 2 out]
              n181 = call "ctl -- name dispatcher.vi"("ctl name dispatch"=ctl_--_name_dispatcher_--_action."peak gamma TEST") -> ("ctl file name"=w373:string)  [unwired: 8 in, 2 out]
              n182 = local read "pm lorentzian"() -> (w403:T5)
              n183 = call "ctl -- name dispatcher.vi"("ctl name dispatch"=ctl_--_name_dispatcher_--_action."peak freq gamma TEST") -> ("ctl file name"=w371:string)  [unwired: 8 in, 2 out]
              n184 = call "file -- 9w path.vi"("sweep folder"=w398) -> ("9w path"=w387:path)  [unwired: 10 in]
              n185 = Unbundle By Name(w403) -> ("omega(0)"=w402:dbl, "Gamma"=w401:dbl)
              n186 = Build Path(base path=w387, name or relative path=w371) -> (appended path=w377:path)
              n187 = Build Path(base path=w387, name or relative path=w373) -> (appended path=w389:path)
              n188 = Build Path(base path=w387, name or relative path=w375) -> (appended path=w397:path)
              n189 = call "Q -- check range -- i -- real.vi"("lower"=w400, "default"=1.0, "number"=w401) -> ("number in range"=w388:dbl)  [unwired: 6 in, 2 out]
              n190 = call "Q -- check range -- i -- real.vi"("lower"=w400, "default"=w400, "number"=w402) -> ("number in range"=w395:dbl)  [unwired: 6 in, 2 out]
              n191 = Number To Fractional String(number=w388) -> (F-format string=w382:string)  [unwired: 3 in]
              n192 = Number To Fractional String(number=w395) -> (F-format string=w383:string)  [unwired: 3 in]
              n193 = Build Array(w382) -> (w391:string[])
              n194 = Build Array(w383) -> (w394:string[])
              n195 = call-poly <vilib>:"Write To Spreadsheet File.vi"("delimiter (\\t)"="\r", "append to file? (new file:F)"=TRUE, "1D data"=w391, "file path (dialog if empty)"=w389) -> ()  [unwired: 4 in, 1 out]
              n196 = call-poly <vilib>:"Write To Spreadsheet File.vi"("delimiter (\\t)"="\r", "append to file? (new file:F)"=TRUE, "1D data"=w394, "file path (dialog if empty)"=w397) -> ()  [unwired: 4 in, 1 out]
              n197 = Concatenate Strings(w383, "\t", w382) -> (w381:string)
              n198 = Build Array(w381) -> (w385:string[])
              n199 = call-poly <vilib>:"Write To Spreadsheet File.vi"("delimiter (\\t)"="\r", "append to file? (new file:F)"=TRUE, "1D data"=w385, "file path (dialog if empty)"=w377) -> ()  [unwired: 4 in, 1 out]
            }
          }
        }
      }
      event Timeout {
        n200 = event-data() -> ()  [unwired: 1 in, 2 out]
      }
    }
    n201 = Wait (ms)(milliseconds to wait=u32 111) -> ()  [unwired: 1 out]
  }
  n202 = Create User Event(user event datatype=w27) -> (user event=w26:refnum<user-event>)  [unwired: 1 in, 1 out]
  n203 = register-events(w26) -> (reference out=w28:refnum<event-registration>)  [unwired: 2 in, 1 out]
  n204 = while {
    tunnel: w28 -> [w411]
    tunnel: w25 -> [w410]
    stop <- FALSE stop-if-true
    n205 = control-ref of="Plot: complex plane"() -> (w404:refnum<vi>)
    n206 = local read "good lorentzian"() -> (w405:T5)
    n207 = local read "cp lorentzian"() -> (w407:T5)
    n208 = control-ref of="cursor bracket: All, data window"() -> (w406:refnum<vi>)
    n209 = event shown="[1] Key Down" {
      selector: w411 -> [_ _ _ _ _ _ _ _ _ _]
      dyn-events: _ -> [_ _ _ _ _ _ _ _ _ _]
      timeout: _ -> [_ _ _ _ _ _ _ _ _ _]
      tunnel: w410 -> [_ w418 _ _ _ _ _ w535 _ _]
      tunnel: w406 -> [_ w417 _ _ _ _ w533 _ _ _]
      tunnel: w407 -> [_ w413 _ _ _ _ _ _ _ w553]
      tunnel: w404 -> [_ w412 _ _ _ _ _ _ _ w551]
      tunnel: w405 -> [_ _ _ _ _ _ _ _ w540 _]
      event Timeout {
        n210 = event-data() -> ()  [unwired: 1 in, 2 out]
      }
      event Key Down {
        n211 = event-data() -> ("Char"=w415:i16, "VKey"=w419:T12)  [unwired: 1 in]
        "Char" <- w415
        "VKey" <- w419
        n212 = Build Array(w415) -> (w416:i16[])
        n213 = Byte Array To String(unsigned byte array=w416) -> (string=w414:string)
        n214 = case shown="\"ASCII\", Default" w419 {
          selector: w419 -> [_ _ _ _ w486]
          tunnel: w415 -> [_ _ _ _ _]
          tunnel: w418 -> [w424 _ w480 w482 w485]
          tunnel: w417 -> [w423 _ _ _ w487]
          tunnel: w414 -> [w422 _ _ _ _]
          tunnel: w413 -> [w421 _ _ _ _]
          tunnel: w412 -> [w420 _ _ _ _]
          frame "ASCII", Default {
            n215 = case shown="\" \"" w422 {
              tunnel: w424 -> [_ _ _ w435 w437 _ _ w443 _ w449 w451 w453 _ w466 w468 w470 w474 w477]
              tunnel: w423 -> [_ _ w432 _ _ w438 w440 _ _ _ _ _ _ _ _ _ _ _]
              tunnel: w421 -> [_ _ _ _ _ _ _ _ _ _ _ _ w454 _ _ _ _ _]
              tunnel: w420 -> [_ _ _ _ _ _ _ _ _ _ _ _ w455 _ _ _ _ _]
              frame "0", Default {
              }
              frame "*" {
                # "*"
                n216 = local read "overwrite (d)"() -> (w427:enum16{"DUMP", "WORK", ""})
                n217 = case shown="\"DUMP\", Default" w427 {
                  tunnel: [enum16{"DUMP", "WORK", ""}."WORK" ("overwrite dump/work (\"d\")") enum16{"DUMP", "WORK", ""}."DUMP" ("overwrite dump/work (\"d\")")] -> w426
                  tunnel: [TRUE ("overwriting !!") FALSE ("overwriting !!")] -> w425
                  frame "DUMP", Default {
                  }
                  frame "WORK" {
                  }
                }
                n218 = local write "overwrite (d)"(w426) -> ()
                n219 = local write "overwriting !!"(w425) -> ()
              }
              frame "?" {
                # "?"
                n220 = call "cursor window logic V2.vi"("cursor window action"=cursor_window_action."zoom X", "cursor window in"=w432) -> ()  [unwired: 8 in, 2 out]
              }
              frame "o" {
                # "o"
                n221 = Generate User Event(user event=w435, event data cluster="calc:new file" ("event data")) -> ()  [unwired: 2 in, 2 out]
              }
              frame "\\" {
                # "\\"
                n222 = Generate User Event(user event=w437, event data cluster="jump to a PID peak" ("event data")) -> ()  [unwired: 2 in, 2 out]
              }
              frame "a" {
                # "\"a\" - zoom out"
                n223 = call "cursor window logic V2.vi"("cursor window action"=cursor_window_action."zoom to all data", "cursor window in"=w438) -> ()  [unwired: 8 in, 2 out]
              }
              frame "c" {
                # "\"c\"- for cursor"
                n224 = call "cursor window logic V2.vi"("cursor window action"=cursor_window_action."check", "cursor window in"=w440) -> ()  [unwired: 8 in, 2 out]
              }
              frame "d" {
                # "d"
                n225 = Generate User Event(user event=w443, event data cluster="dump OLD peak gamma" ("event data")) -> ()  [unwired: 2 in, 2 out]
              }
              frame "e" {
                # "e"
                n226 = local read "Tab : monitor"() -> (w445:enum32{"main", "EDIT"})
                n227 = case shown="\"main\", Default" w445 {
                  tunnel: [enum32{"main", "EDIT"}."EDIT" ("Tab : monitor") enum32{"main", "EDIT"}."main" ("Tab : monitor")] -> w444
                  frame "main", Default {
                  }
                  frame "EDIT" {
                  }
                }
                n228 = local write "Tab : monitor"(w444) -> ()
              }
              frame "n" {
                n229 = Generate User Event(user event=w449, event data cluster="dump NEW peak gamma" ("event data")) -> ()  [unwired: 2 in, 2 out]
              }
              frame "q" {
                # "n"
                n230 = Generate User Event(user event=w451, event data cluster="save search window" ("event data")) -> ()  [unwired: 2 in, 2 out]
              }
              frame "Q" {
                n231 = Generate User Event(user event=w453, event data cluster="save current lorentzian" ("event data")) -> ()  [unwired: 2 in, 2 out]
              }
              frame " " {
                n232 = Unbundle By Name(w454) -> ("4corners.z center"=w463:cdb)
                n233 = local read "scale gauge: Plot: complex plane"() -> (w464:dbl)
                n234 = Complex To Re/Im(x + iy=w463) -> (x=w462:dbl, y=w461:dbl)
                n235 = Negate(x=w464) -> (-x=w456:dbl)
                n236 = Add(x=w461, y=w456) -> (x+y=w460:dbl)
                n237 = Add(x=w462, y=w456) -> (x+y=w457:dbl)
                n238 = Add(x=w461, y=w464) -> (x+y=w459:dbl)
                n239 = Add(x=w462, y=w464) -> (x+y=w458:dbl)
                n240 = property on="Property Node" class="XYGraph (strict)"(reference=w455, "XScale.Minimum"=w457, "XScale.Maximum"=w458, "YScale.Maximum"=w459, "YScale.Minimum"=w460) -> ()  [unwired: 1 in, 2 out]
              }
              frame "y" {
                # "y"
                n241 = Generate User Event(user event=w466, event data cluster="append a line" ("event data")) -> ()  [unwired: 2 in, 2 out]
              }
              frame "I" {
                # "y"
                n242 = Generate User Event(user event=w468, event data cluster="insert resonance -- from window" ("event data")) -> ()  [unwired: 2 in, 2 out]
              }
              frame "R" {
                # "y"
                n243 = Generate User Event(user event=w470, event data cluster="delete resonance" ("event data")) -> ()  [unwired: 2 in, 2 out]
              }
              frame "U" {
                n244 = for {
                  N: 100 -> [_]
                  tunnel: [w475] -> w471 mode=indexing
                  i -> [w475]
                }
                "index" <- w471
                n245 = Generate User Event(user event=w474, event data cluster="reread resonances" ("event data")) -> ()  [unwired: 2 in, 2 out]
              }
              frame "v" {
                # "v"
                n246 = Generate User Event(user event=w477, event data cluster="scan for existing peaks" ("event data")) -> ()  [unwired: 2 in, 2 out]
              }
            }
          }
          frame "Escape" {
            n247 = local read "use fast fit?"() -> (w478:bool)
            n248 = Not(x=w478) -> (.not. x?=w479:bool)
            n249 = local write "use fast fit?"(w479) -> ()
          }
          frame "PageUp" {
            n250 = Generate User Event(user event=w480, event data cluster="next resonance" ("event data")) -> ()  [unwired: 2 in, 2 out]
          }
          frame "PageDown" {
            n251 = Generate User Event(user event=w482, event data cluster="prev resonance" ("event data")) -> ()  [unwired: 2 in, 2 out]
          }
          frame "Up".."Right" {
            n252 = case shown="\"Left\"" w486 {
              tunnel: w487 -> [w488 w490 w492 w495]
              frame "Right", Default {
                n253 = call "cursor window logic V2.vi"("cursor window action"=cursor_window_action."move right", "cursor window in"=w488) -> ()  [unwired: 8 in, 2 out]
              }
              frame "Left" {
                n254 = call "cursor window logic V2.vi"("cursor window action"=cursor_window_action."move left", "cursor window in"=w490) -> ()  [unwired: 8 in, 2 out]
              }
              frame "Up" {
                n255 = call "cursor window logic V2.vi"("cursor window action"=cursor_window_action."broaden", "cursor window in"=w492) -> ()  [unwired: 8 in, 2 out]
              }
              frame "Down" {
                n256 = call "cursor window logic V2.vi"("cursor window action"=cursor_window_action."shrink", "cursor window in"=w495) -> ()  [unwired: 8 in, 2 out]
              }
            }
            n257 = Generate User Event(user event=w485, event data cluster="one peak" ("event data")) -> ()  [unwired: 2 in, 2 out]
          }
        }
      }
      event Value Change {
        n258 = event-data() -> ("CtlRef"=w499:refnum<vi>)  [unwired: 1 in, 5 out]
        n259 = local read "scan monitor control"() -> (w497:T1)
        n260 = property class="Ctl"(reference=w499) -> ("Label.Text"=w498:string)  [unwired: 1 in, 2 out]
        n261 = case shown="\"Unique strike pars\", Default" w498 {
          tunnel: w497 -> [w501 w512]
          tunnel: [w500 w511] -> w496
          frame "Unique strike pars", Default {
            n262 = in-place {
              n263 = in-place-cluster #5(w501) -> ("Unique strike parameters"=w505:bool)  [unwired: 1 out]
              n264 = Not(x=w505) -> (.not. x?=w504:bool)
              n265 = case shown="True" w504 {
                selector: w504 -> [w508 w509]
                tunnel: [enum16{"funnel open", "funnel closed"}."funnel open" ("funnel state") enum16{"funnel open", "funnel closed"}."funnel closed" ("funnel state")] -> w506
                tunnel: [w508 w509] -> w503
                frame False {
                }
                frame True {
                }
              }
              n266 = Not(x=w503) -> (.not. x?=w502:bool)
              n267 = in-place-cluster #5("Unique strike parameters"=w502, "funnel state"=w506) -> (w500:T1)
            }
          }
          frame "funnel state" {
            n268 = in-place {
              n269 = in-place-cluster #6(w512) -> ("funnel state"=w515:enum16{"funnel open", "funnel closed"})  [unwired: 1 out]
              n270 = case shown="\"funnel closed\"" w515 {
                selector: w515 -> [w518 w520]
                tunnel: [w518 w520] -> w516
                tunnel: [FALSE TRUE] -> w513
                frame "funnel open", Default {
                }
                frame "funnel closed" {
                }
              }
              n271 = Not(x=w513) -> (.not. x?=w514:bool)
              n272 = in-place-cluster #6("Unique strike parameters"=w514, "funnel state"=w516) -> (w511:T1)
            }
          }
        }
        n273 = local write "scan monitor control"(w496) -> ()
      }
      event "use fast fit?": Value Change {
        n274 = event-data() -> ()  [unwired: 1 in, 6 out]
      }
      event "overwrite (d)": Value Change {
        n275 = event-data() -> ("NewVal"=w522:enum16{"DUMP", "WORK", ""})  [unwired: 1 in]
        n276 = case shown="\"DUMP\", Default" w522 {
          tunnel: [FALSE ("overwriting !!") TRUE ("overwriting !!")] -> w521
          frame "DUMP", Default {
          }
          frame "WORK" {
          }
        }
        n277 = local write "overwriting !!"(w521) -> ()
      }
      event "autopilot": Value Change {
        n278 = event-data() -> ("NewVal"=w527:enum32{"on", "off"})  [unwired: 1 in]
        n279 = local read "scan monitor control"() -> (w526:T1)
        n280 = case shown="\"on\"" w527 {
          tunnel: w526 -> [w530 w531]
          tunnel: [w528 w531] -> w525
          frame "on" {
            n281 = Bundle By Name(cluster=w530, "overwrite ctl?"=TRUE ("overwrite?")) -> (w528:T1)
          }
          frame "off", Default {
          }
        }
        n282 = local write "scan monitor control"(w525) -> ()
      }
      event "Plot: All": Cursor Move {
        n283 = event-data() -> ("CursIdx"=w532:i32)  [unwired: 1 in, 3 out]
        n284 = call "cursor window logic V2.vi"("CursIdx"=w532, "cursor window action"=cursor_window_action."cursor moves", "cursor window in"=w533) -> ()  [unwired: 7 in, 2 out]
      }
      event "Plot: All": Cursor Release {
        n285 = event-data() -> ("CursIdx"=w536:i32)  [unwired: 1 in, 3 out]
        n286 = case shown="0..2" w536 {
          tunnel: w535 -> [_ w537]
          frame 3, Default {
          }
          frame 0..2 {
            w538 = "one peak"  # event data
            n287 = Generate User Event(user event=w537, event data cluster=w538) -> ()  [unwired: 2 in, 2 out]
          }
        }
      }
      event "scale gauge: Plot: complex plane - filter": Value Change {
        n288 = event-data() -> ("NewVal"=w542:dbl)  [unwired: 1 in]
        n289 = Unbundle By Name(w540) -> ("4corners.z center"=w541:cdb)
        n290 = Unbundle By Name(w540) -> ("4corners"=→"4corners":T6)
        n291 = Complex To Re/Im(x + iy=w541) -> (x=w544:dbl, y=w545:dbl)
        n292 = Negate(x=w542) -> (-x=w550:dbl)
        n293 = control-ref of="Plot: complex plane - filter"() -> (w543:refnum<vi>)
        n294 = Add(x=w545, y=w550) -> (x+y=w546:dbl)
        n295 = Add(x=w544, y=w542) -> (x+y=w548:dbl)
        n296 = Add(x=w544, y=w550) -> (x+y=w549:dbl)
        n297 = Add(x=w545, y=w542) -> (x+y=w547:dbl)
        n298 = property on="Property Node" class="XYGraph (strict)"(reference=w543, "XScale.Minimum"=w549, "XScale.Maximum"=w548, "YScale.Maximum"=w547, "YScale.Minimum"=w546) -> ()  [unwired: 1 in, 2 out]
      }
      event "scale gauge: Plot: complex plane": Value Change {
        n299 = event-data() -> ("NewVal"=w554:dbl)  [unwired: 1 in]
        n300 = Unbundle By Name(w553) -> ("4corners.z center"=w552:cdb)
        n301 = Complex To Re/Im(x + iy=w552) -> (x=w555:dbl, y=w556:dbl)
        n302 = Negate(x=w554) -> (-x=w561:dbl)
        n303 = Add(x=w556, y=w561) -> (x+y=w557:dbl)
        n304 = Add(x=w555, y=w554) -> (x+y=w559:dbl)
        n305 = Add(x=w555, y=w561) -> (x+y=w560:dbl)
        n306 = Add(x=w556, y=w554) -> (x+y=w558:dbl)
        n307 = property on="Property Node" class="XYGraph (strict)"(reference=w551, "XScale.Minimum"=w560, "XScale.Maximum"=w559, "YScale.Maximum"=w558, "YScale.Minimum"=w557) -> ()  [unwired: 1 in, 2 out]
      }
    }
    n308 = Wait (ms)(milliseconds to wait=u32 31) -> ()  [unwired: 1 out]
  }
  n309 = control-ref of="timer \"v\""() -> (w24:refnum<vi>)
  n310 = control-ref of="timer  \"update\""() -> (w7:refnum<vi>)
  n311 = call "slider timer .vi"("action"=w6, "timer ref"=w7) -> ("timer out"=w5:refnum<vi>)  [unwired: 7 in, 2 out]
  n312 = call "slider timer .vi"("action"=w6, "timer ref"=w24) -> ("timer out"=w3:refnum<vi>)  [unwired: 7 in, 2 out]
  n313 = local read "file path"() -> (w4:path)
  n314 = call "slider timer .vi"("action"=countdown_control."stop", "timer ref"=w3) -> ("timer out"=w2:refnum<vi>)  [unwired: 7 in, 2 out]
  n315 = while {
    tunnel: w25 -> [w573]
    shift-right: [w577] -> _
    shift-left: w2 -> [w578]
    shift-right: [w571] -> _
    shift-left: w5 -> [w572]
    shift-right: [w568] -> _
    shift-left: w4 -> [w569]
    stop <- FALSE stop-if-true
    (unwired) 0
    n316 = case shown="\"on\"" "autopilot" {
      tunnel: [FALSE TRUE] -> w563
      frame "off", Default {
      }
      frame "on" {
      }
    }
    n317 = call "slider timer .vi"("action"=countdown_control."check", "timer ref"=w572) -> ("tic"=w567:bool, "timer out"=w571:refnum<vi>)  [unwired: 7 in, 1 out]
    n318 = Compound Arithmetic op=AND(w567, w563) -> (w566:bool)
    n319 = case shown="True" w566 {
      tunnel: w569 -> [w586 w590]
      tunnel: [w586 w588] -> w568
      tunnel: [FALSE w587] -> w562
      frame False {
      }
      frame True {
        n320 = local read "Sweep folder path"() -> (w595:path)
        n321 = call "latest scan file.vi"("source"=enum16{"last scan file", "manual"}."last scan file", "file path in"=w590, "sweep folder"=w595) -> ("temperature (K)"=w594:dbl, "file or folder exists?"=w589:bool, "file path out"=w591:path)  [unwired: 5 in, 1 out]
        n322 = Not Equal?(x=w591, y=w590) -> (x != y?=w592:bool)
        n323 = And(x=w589, y=w592) -> (x .and. y?=w587:bool)
        n324 = local write "Temperature (K)"(w594) -> ()
        n325 = Select(t=w591, s=w587, f=w590) -> (s? t:f=w588:path)
        n326 = local write "file path"(w588) -> ()
        n327 = local write "scan file found"(w589) -> ()
      }
    }
    n328 = Wait (ms)(milliseconds to wait=u32 123) -> ()  [unwired: 1 out]
    n329 = Select(t=countdown_control."reset once" ("action"), s=w562, f=countdown_control."check" ("action")) -> (s? t:f=w574:T16)
    n330 = call "slider timer .vi"("action"=w574, "timer ref"=w578) -> ("tic"=w565:bool, "timer out"=w577:refnum<vi>)  [unwired: 7 in, 1 out]
    n331 = And(x=w563, y=w565) -> (x .and. y?=w579:bool)
    n332 = case shown="True" w579 {
      tunnel: w573 -> [_ w596]
      frame False {
      }
      frame True {
        w597 = "scan for existing peaks"  # calculate
        n333 = Generate User Event(user event=w596, event data cluster=w597) -> ()  [unwired: 2 in, 2 out]
      }
    }
    n334 = And(x=w563, y=w562) -> (x .and. y?=w580:bool)
    n335 = case shown="True" w580 {
      tunnel: w573 -> [_ w599]
      frame False {
      }
      frame True {
        w598 = "calc:new file"  # calculate
        n336 = Generate User Event(user event=w599, event data cluster=w598) -> ()  [unwired: 2 in, 2 out]
      }
    }
  }
